vi "edit IPF.vi"(0 "New IPF":bool, 1 "Programs List":i32, 2 "APG Config":T6={"IPF Folder"=path "", "Results Folder"=path "", "Trace Folder"=path "", "a3DiCAD"={"Plot Spacing"=0.0, "TCF"=enum."STANDARD", "LeadLimit"=0, "a3DiCADDebug"=FALSE, "ODB"={"PrimePartNumber"=[], "SecondPartNumber"=[], "Height"={"PRP_CMP"="", "HEIGHT"=""}, "Units"={"PRP_CMP"="", "UNITS"=""}}, "PasteHeight"=0.0, "Inspection Performance"=TRUE}, "a3DiCADcfg"=path "", "Board Library"={"Board Library file"=path "", "Board library model folder"=path "", "Not Fittted/Fitted Components"=path "", "Panel Picture File"=path "", "Components"=enum."Fitted"}, "Site Library"={"Site Library file"=path "", "Site library model folder"=path ""}, "System Library"={"System Library file"=path "", "System library model folder"=path ""}, "ODB++ file"=path "", "Side ID Alias"={"Top"="", "Bottom"=""}}, 3 "Dongle Fitted event Refnum in":T1, 5 "error in":errorcluster, 6 "Main VI":refnum<vi>) -> (14 "Dongle fitted":bool, 16 "Program Name":string, 19 "error out":errorcluster)   [LabVIEW 2013, in "Manipulate IPF.lvlib"]
uses:
  Manipulate IPF.lvlib
  type_def/but_back.ctl
  3013/code/Modules/Configuration/type_def/Scan Params.ctl
  3013/code/Modules/Configuration/type_def/Profile Resolution.ctl
  3013/code/Modules/Preprocess Data/type_def/direction.ctl
  3013/code/Modules/GUI/GUI_5/subPanels/edit/type_def/GUI PCB List.ctl
  3013/code/Modules/Inspection/Data/PCB_class/type_def/PCB Params.ctl
  3013/code/Modules/Inspection/type_def/Pos and Rot.ctl
  3013/code/Modules/Barcode Reader/type_def/id.ctl
  3013/code/Modules/GUI/GUI_5/subPanels/edit/type_def/GUI Panel Params.ctl
  3013/code/Modules/Inspection/type_def/Range Limits.ctl
  3013/code/Modules/GUI/GUI_5/subPanels/edit/type_def/Description.ctl
  Settings/type_def/APG Config.ctl
  type_def/but_debug.ctl
  type_def/but_update TCF.ctl
  type_def/but_test coverage.ctl
  type_def/but_generate_Library_from TCF.ctl
  type_def/Dongle fitted event refnum.ctl
  type_def/state.ctl
  type_def/files.ctl
  3013/code/Modules/Inspection/Data/Panel_class/type_def/Config File data.ctl
  3013/code/Modules/Inspection/Data/Panel_class/type_def/BarCode Params.ctl
  3013/code/Modules/GUI/GUI_5/subPanels/edit/type_def/data.ctl
  3013/code/Modules/Inspection/Data/Panel_class/type_def/inspection data.ctl
  <vilib>/Utility/miscctls.llb/LVFontTypeDef.ctl
  type_def/Picture FGV commands.ctl
  Pack Data/type_def/file types.ctl
  type_def/IPF cmd.ctl
  <userlib>/_OpenG.lib/file/file.llb/Convert File Extension (Path)__ogtk.vi
  <userlib>/_OpenG.lib/file/file.llb/Strip Path Extension - 1D Array of Strings__ogtk.vi
  <userlib>/_OpenG.lib/file/file.llb/File Exists - Scalar__ogtk.vi
  <vilib>/Utility/cursorutil.llb/Set Cursor (Icon Pict).vi
  a3Di APG.lvlib
  3013/code/Modules/Inspection/Inspection.lvlib
  3013/code/Modules/Inspection/Data/PCB_class/PCB.lvclass
  3013/code/Modules/Barcode Reader/Barcode Reader.lvlib
  3013/code/Modules/Inspection/Data/Panel_class/Panel.lvclass
  3013/code/Modules/GUI/GUI_5/subPanels/edit/edit.lvlib
  3013/code/Modules/Preprocess Data/PreProcess.lvlib
  3013/code/Modules/Configuration/Config.lvlib
  Debug Results/Debug Results.lvlib
  3013/code/a3Di.lvlib
  Pack Data/Pack Files.lvlib
  3013/code/Modules/Inspection/Data/Fiducial_class/Fiducial.lvclass
  Mike/APG_mike a3Di.lvlib
  Update TCF/TCF update.lvlib
  Settings/APG_settings.lvlib
panel:
  in  "Side ID":string(combo)
  in  "Product Code":string
  in  "Initial Scan Button":bool caption="Initial Scan"
  in  "Generate Library button":T2
  in  "Test Coverage Button":T3
  in  "Update CAD Picture":bool
  in  "Delete CAD Picture":bool
  out "Panel Picture File":string
  in  "Update TCF button":T4
  out "PCB Outline File":string
  out "Control File":string
  out "Checking results":string
  in  "Debug Results Button":T5
  in  "Start Conversion ODB++":bool
  in  "Robot Scan Direction":enum32{"X", "Y", "X and Y"}(radio)
  in  "Add Fiducial":bool
  in  "Add PCB":bool
  in  "butReload":bool
  in  "butSave":bool
  in  "Description":T7
  in  "Fiducial List":T10(array[cluster]) {"Fiducial"."Pos & Rot"."Y" format="%#_8g"; "Fiducial"."Pos & Rot"."X" format="%#_8g"}
  in  "PCBs List":T11 {"PCB Params"."Pos & Rot"."Y" format="%#_8g"; "PCB Params"."Pos & Rot"."X" format="%#_8g"}
  in  "Panel Parameters":T14 {"Pos & Rot"."rotation" format="%#.3g"; "Pos & Rot"."Y" format="%#.3g"; "Pos & Rot"."X" format="%#.3g"}
  in  "Scan Params":T15={"Size of Scanning Area"={"x"=164.0, "y"=70.0}, "Scan Offset"={"x"=164.0, "y"=70.0}, "Slice Step in mm"=10.0, "Triggering Distance in mm"=0.0, "Triggering Distance in um"=0.0, "Profile Resolution"=enum."20 um", "Version"="", "Robot Scan Direction"=enum."X", "Initial scan"=FALSE}
  out "Program Name":string
  in  "Back Button":T18
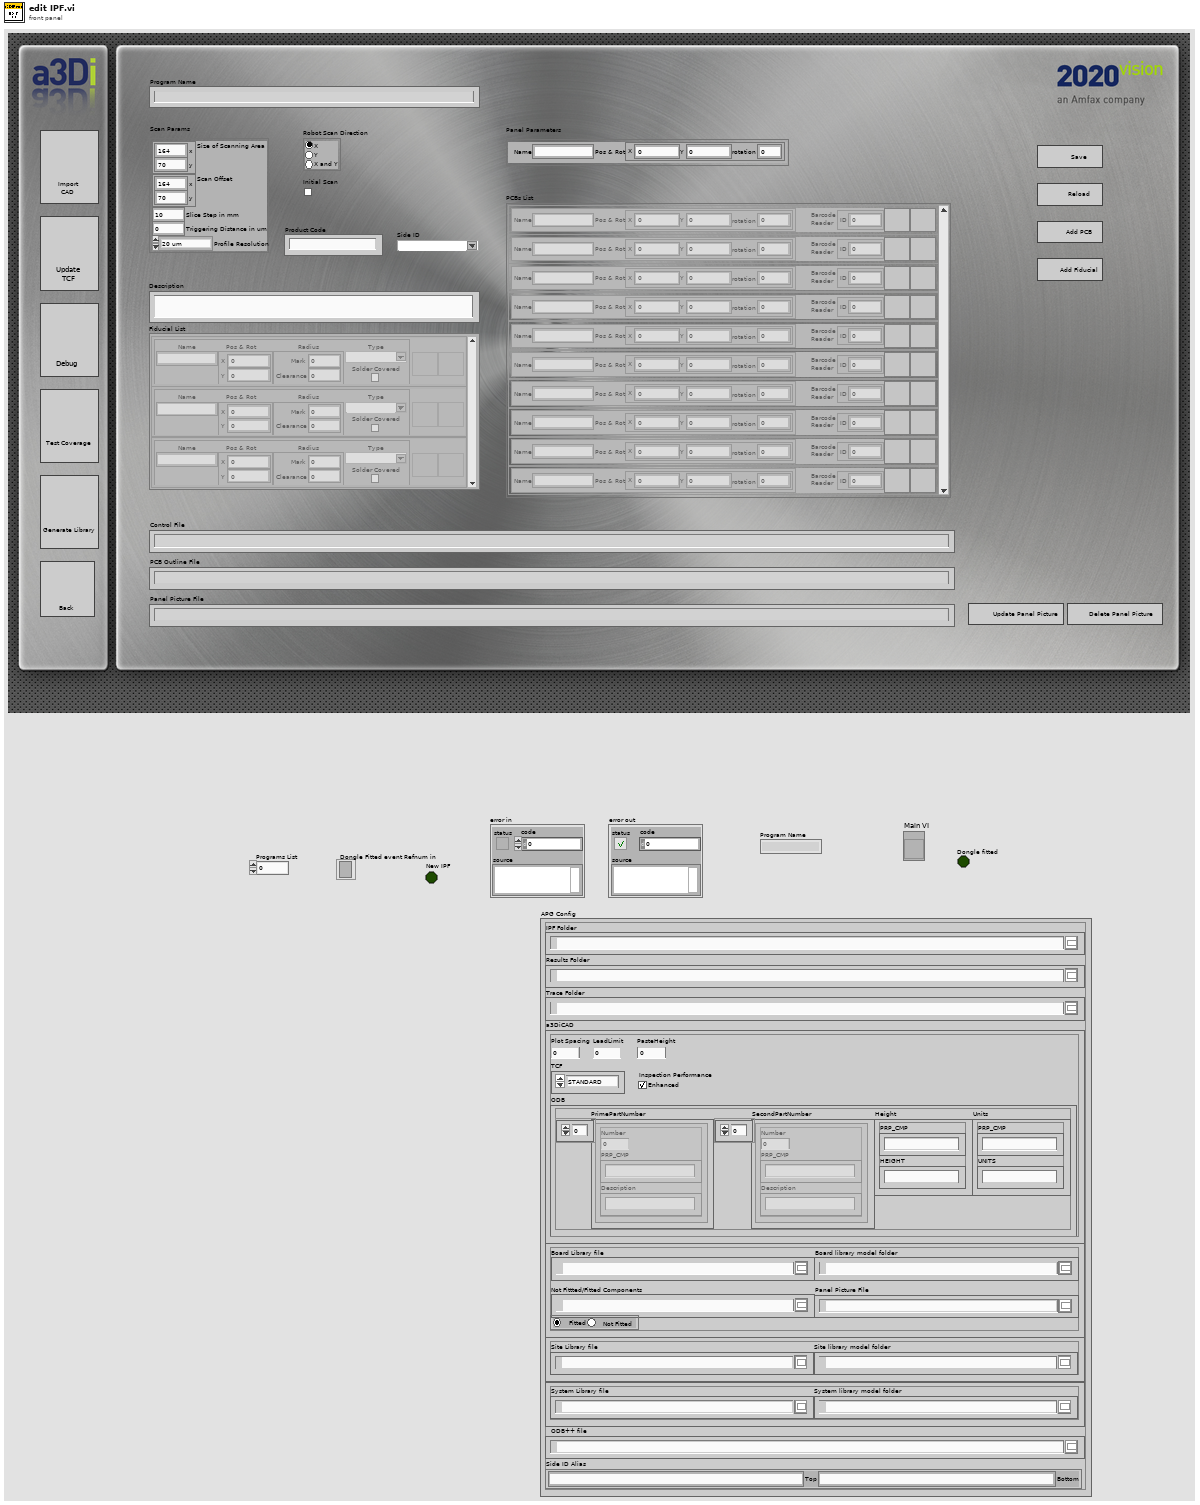
[diagram p1: front panel]
types:
  T1 = typedef "Dongle fitted event refnum.ctl" = refnum<event-registration>
  T2 = typedef "but_generate_Library_from TCF.ctl" = bool
  T3 = typedef "but_test coverage.ctl" = bool
  T4 = typedef "a3Di APG.lvlib/but_update TCF.ctl" = bool
  T5 = typedef "but_debug.ctl" = bool
  T6 = typedef "APG_settings.lvlib/APG Config.ctl" = cluster{"IPF Folder":path, "Results Folder":path, "Trace Folder":path, "a3DiCAD":cluster{"Plot Spacing":dbl, "TCF":enum16{"STANDARD", "PASTE", "LEAD"}, "LeadLimit":u32, "a3DiCADDebug":bool, "ODB":cluster{"PrimePartNumber":cluster{"Number":u32, "PRP_CMP":string, "Description":string}[], "SecondPartNumber":cluster{"Number":u32, "PRP_CMP":string, "Description":string}[], "Height":cluster{"PRP_CMP":string, "HEIGHT":string}, "Units":cluster{"PRP_CMP":string, "UNITS":string}}, "PasteHeight":dbl, "Inspection Performance":bool}, "a3DiCADcfg":path, "Board Library":cluster{"Board Library file":path, "Board library model folder":path, "Not Fittted/Fitted Components":path, "Panel Picture File":path, "Components":enum32{"Fitted", "Not Fitted "}}, "Site Library":cluster{"Site Library file":path, "Site library model folder":path}, "System Library":cluster{"System Library file":path, "System library model folder":path}, "ODB++ file":path, "Side ID Alias":cluster{"Top":string, "Bottom":string}}
  T7 = typedef "Description.ctl" = string
  T8 = typedef "Inspection.lvlib/Pos and Rot.ctl" = cluster{"X":dbl, "Y":dbl, "Z":dbl, "rotation":dbl}
  T9 = typedef "Inspection.lvlib/Range Limits.ctl" = cluster{"upper":sgl, "lower":sgl}
  T10 = cluster{"Fiducial":cluster{"Name":string, "Pos & Rot":T8, "Radius":cluster{"Mark":dbl, "Clearance":dbl}, "Inspection Params":cluster{"Clearance vs\nPad Threshold":dbl, "Avg Plane Limits":T9, "Edge Limit":T9}, "Type":string, "Solder Covered":bool}, "insert":bool, "delete":bool}[]
  T11 = typedef "GUI.lvlib/subPanel.lvlib/edit.lvlib/GUI PCB List.ctl" = cluster{"PCB Params":T12, "Barcode\nReader":cluster{"ID":T13}, "insert":bool, "delete":bool}[]
  T12 = typedef "Inspection.lvlib/PCB.lvclass/PCB Params.ctl" = cluster{"Name":string, "Pos & Rot":T8}
  T13 = typedef "Barcode Reader.lvlib/id.ctl" = u8
  T14 = typedef "GUI.lvlib/subPanel.lvlib/edit.lvlib/GUI Panel Params.ctl" = cluster{"Name":string, "Pos & Rot":T8}
  T15 = typedef "Config.lvlib/Scan Params.ctl" = cluster{"Size of Scanning Area":cluster{"x":dbl, "y":dbl}, "Scan Offset":cluster{"x":dbl, "y":dbl}, "Slice Step in mm":dbl, "Triggering Distance in mm":dbl, "Triggering Distance in um":dbl, "Profile Resolution":T16, "Version":string, "Robot Scan Direction":T17, "Initial scan":bool}
  T16 = typedef "Config.lvlib/Profile Resolution.ctl" = enum8{"20 um", "40 um"}
  T17 = typedef "PreProcess.lvlib/direction.ctl" = enum8{"X", "Y"}
  T18 = typedef "a3Di APG.lvlib/but_back.ctl" = bool
  T19 = typedef "GUI.lvlib/subPanel.lvlib/edit.lvlib/data.ctl" = cluster{"Program Name":string, "Scan Params[]":T15[], "Panel Params":T20, "Inspection Data":T22, "Control File Relative Path":path, "Description":string, "PCB Outline File":path, "Scan Start Delay":dbl, "CAD Picture File":string, "Product Code":string, "Side ID":string}
  T20 = typedef "Inspection.lvlib/Panel.lvclass/Config File data.ctl" = cluster{"Name":string, "Pos & Rot":T8, "PCBs List":cluster{"PCB Params":T12}[], "PCB BarCode Params":T21[], "Scan Type":bool}
  T21 = typedef "Inspection.lvlib/Panel.lvclass/BarCode Params.ctl" = cluster{"ID":T13}
  T22 = typedef "Inspection.lvlib/Panel.lvclass/inspection data.ctl" = cluster{"Fiducial List":cluster{"Name":string, "Position and Rotation":T8, "Radius":cluster{"Mark":dbl, "Clearance":dbl}, "Inspection Params":cluster{"Clearance vs Pad\nThreshold":dbl, "Avg Plane Limits":T9, "Edge Limit":T9}, "Type":string, "Solder Covered":bool}[]}
  T23 = typedef "a3Di APG.lvlib/files.ctl" = cluster{"Programming Files":cluster{"PCB Design Identity":string, "ODB++ file":path, "Result temp  folder":path, "IPF temp folder":path}, "ODB file Converted?":bool, "Panel Params":T20, "PCB Outline File":path, "Initial Scan":bool, "PCBs on a carrier":bool, "Carrier Size":cluster{"X":dbl, "Y":dbl}, "IPF modified":bool, "PCB Side":enum16{"Top", "Bottom"}}
  T24 = typedef "Manipulate IPF.lvlib/state.ctl" = enum16{"Initialise Inspection Program", "Wait for user input", "exit"}
  T25 = typedef "Manipulate IPF.lvlib/Picture FGV commands.ctl" = enum16{"No Action", "Set Update Picture", "Set Delete Picture", "Get Picture action"}
  T26 = typedef "LVFontTypeDef.ctl" = cluster{"Font Name":string, "Size":u16, "Bold":bool, "Italic":bool, "Underline":bool, "Strikeout":bool, "Color":u32}
  T27 = enum8{"Enabled", "Disabled", "Disabled and Grayed Out"}
  T28 = typedef "Pack Files.lvlib/file types.ctl" = enum16{"ODB", "TCF", "CAD Outline", "Config", "Inspection Prog", "a3Di-bin", "Results", "CAD Labels", "CAD Pads", "calScan_fid", "calScan_cal-tab", "PCB_SerialNumber", "CAD_Assembly", "Version", "Old Results", "CAD Picture", "Old TCF"}
  T29 = typedef "Manipulate IPF.lvlib/IPF cmd.ctl" = enum16{"New IPF", "Edit IPF", "Copy IPF", "Rename IPF", "Delete IPF", "Reload IPF", "Load all IPF"}
  T30 = cluster{"Debug Results Button":refnum<vi>, "insert":refnum<vi>, "Update TCF button":refnum<vi>, "delete":refnum<vi>, "Test Coverage Button":refnum<vi>, "PCBs List":refnum<vi>, "Fiducial List":refnum<vi>, "Scan Params":refnum<vi>, "Generate Library Button":refnum<vi>}
  T31 = cluster{"PCB Params":T12, "Barcode\nReader":cluster{"ID":T13}, "insert":bool, "delete":bool}
  T32 = cluster{"Fiducial":cluster{"Name":string, "Pos & Rot":T8, "Radius":cluster{"Mark":dbl, "Clearance":dbl}, "Inspection Params":cluster{"Clearance vs\nPad Threshold":dbl, "Avg Plane Limits":T9, "Edge Limit":T9}, "Type":string, "Solder Covered":bool}, "insert":bool, "delete":bool}
  T33 = cluster{"Name":string, "Pos & Rot":T8, "Radius":cluster{"Mark":dbl, "Clearance":dbl}, "Inspection Params":cluster{"Clearance vs\nPad Threshold":dbl, "Avg Plane Limits":T9, "Edge Limit":T9}, "Type":string, "Solder Covered":bool}
  T34 = typedef "Manipulate IPF.lvlib/Picture FGV actions.ctl" = enum16{"No Action", "Update Picture", "Delete Picture"}
  T35 = cluster{"PCB Params":cluster{"Name":bool, "Pos & Rot":cluster{"X":bool, "Y":bool, "Z":bool, "rotation":bool}}, "Barcode\nReader":cluster{"ID":bool}, "insert":bool, "delete":bool}[]
  T36 = cluster{"Fiducial":cluster{"Name":bool, "Pos & Rot":cluster{"X":bool, "Y":bool, "Z":bool, "rotation":bool}, "Radius":cluster{"Mark":bool, "Clearance":bool}, "Inspection Params":cluster{"Clearance vs\nPad Threshold":bool, "Avg Plane Limits":cluster{"upper":bool, "lower":bool}, "Edge Limit":cluster{"upper":bool, "lower":bool}}, "Type":bool, "Solder Covered":bool}, "insert":bool, "delete":bool}[]
  T37 = enum16{"Left", "Centre Left", "Centre Right", "Right", "Panel Close"}
  T38 = typedef "GUI.lvlib/subPanel.lvlib/edit.lvlib/GUI Panel & PCB params.ctl" = cluster{"Panel Params":T14, "PCBs List":T11}
  T39 = typedef "GUI.lvlib/subPanel.lvlib/edit.lvlib/GUI Fiducial List.ctl" = cluster{"Fiducial":cluster{"Name":string, "Pos & Rot":T8, "Radius":cluster{"Mark":dbl, "Clearance":dbl}, "Inspection Params":cluster{"Clearance vs\nPad Threshold":dbl, "Avg Plane Limits":T9, "Edge Limit":T9}, "Type":string, "Solder Covered":bool}, "insert":bool, "delete":bool}[]
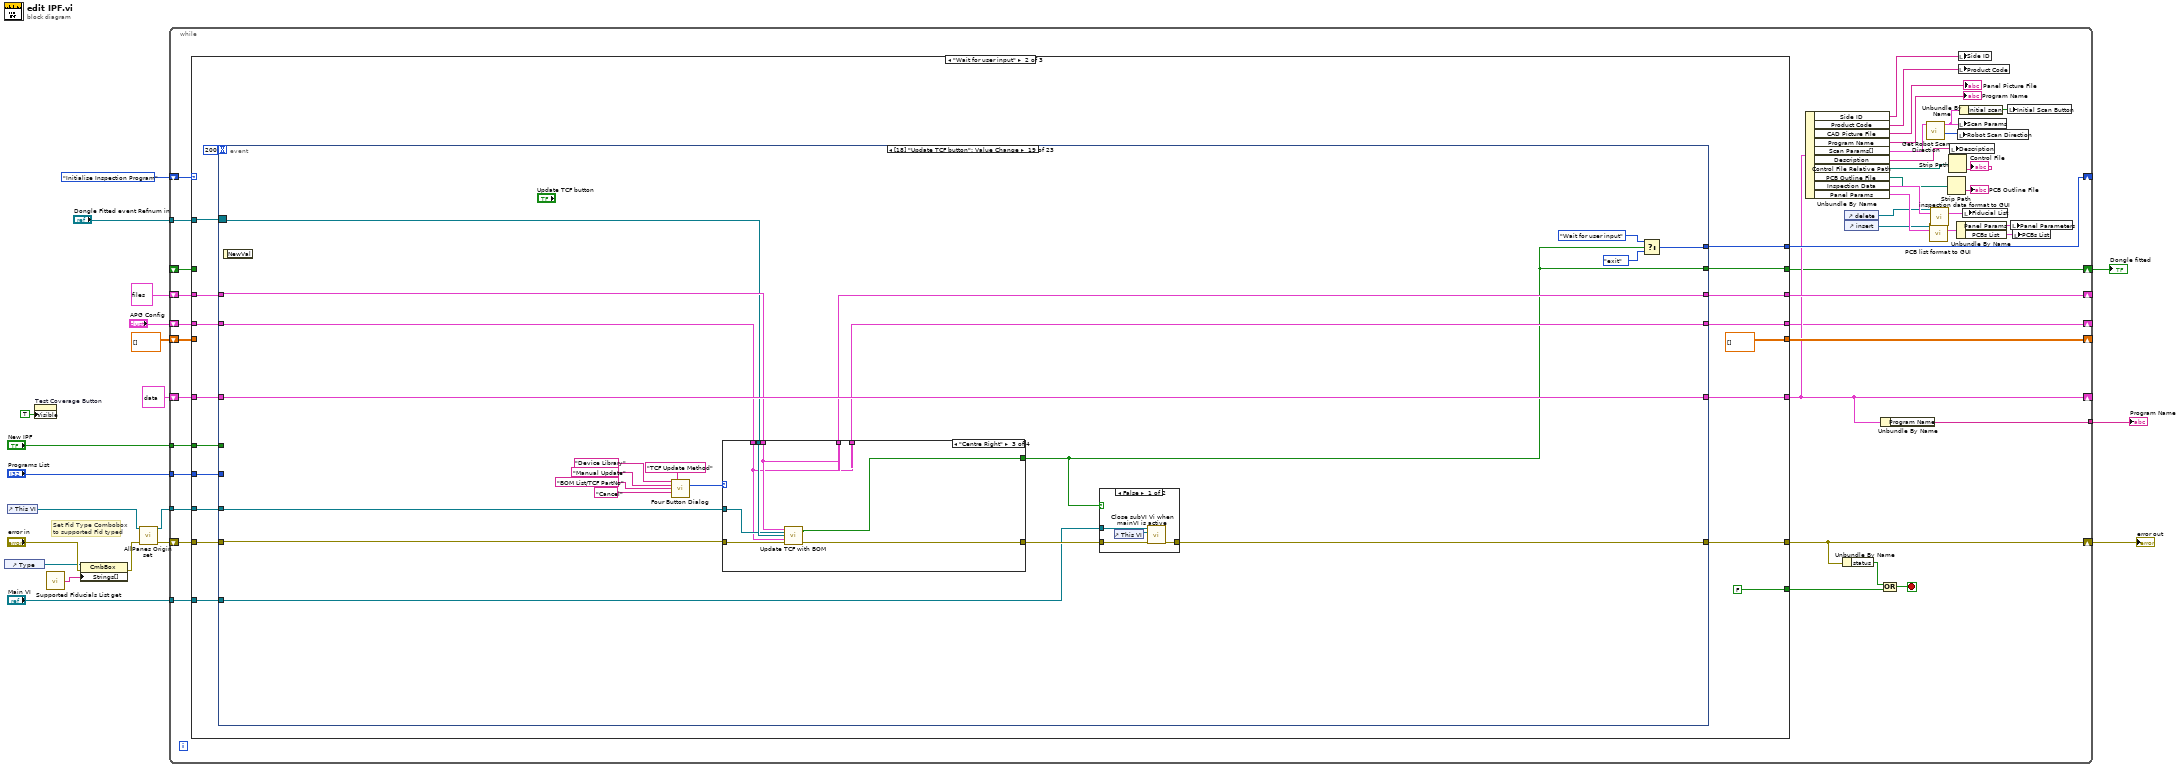
[diagram p0: block diagram]
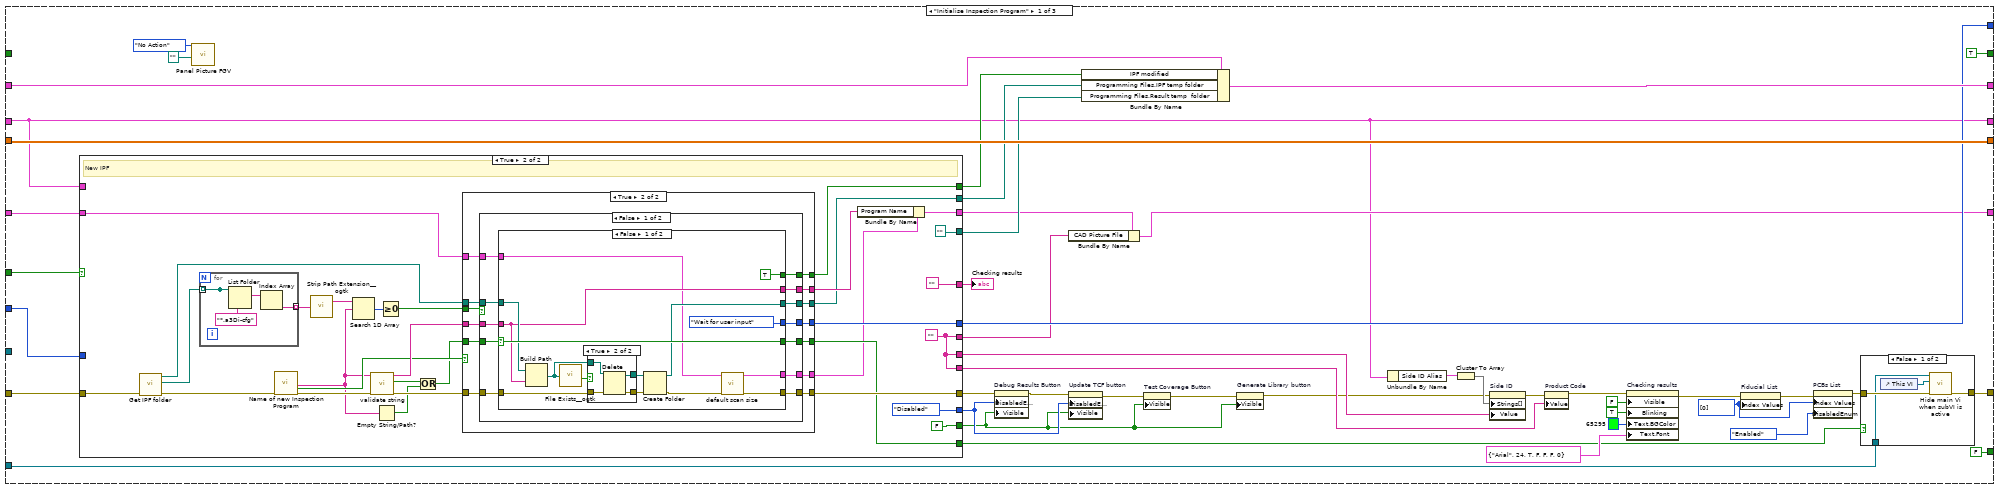
[diagram p2: hidden frame]
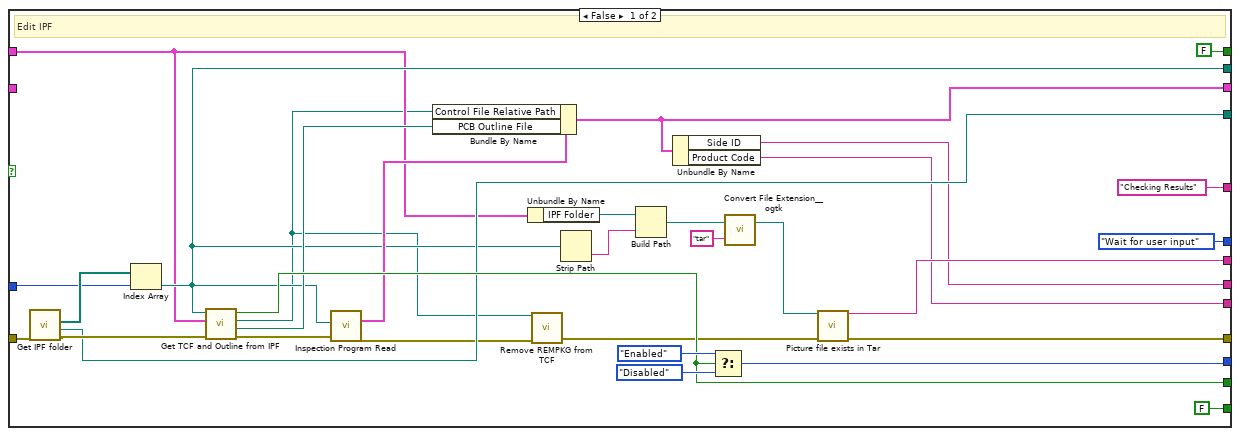
[diagram p4: hidden frame]
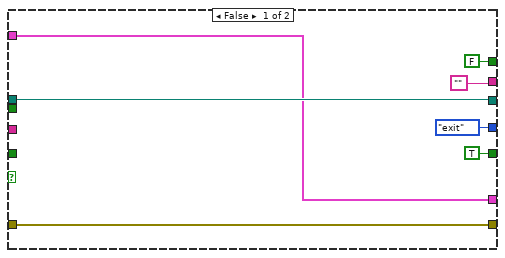
[diagram p5: hidden frame]
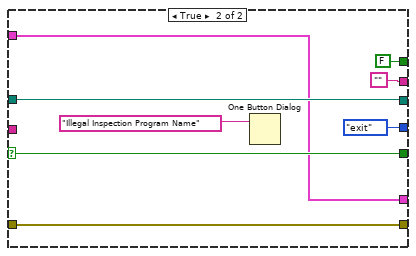
[diagram p7: hidden frame]
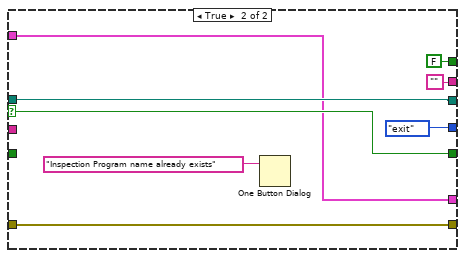
[diagram p8: hidden frame]
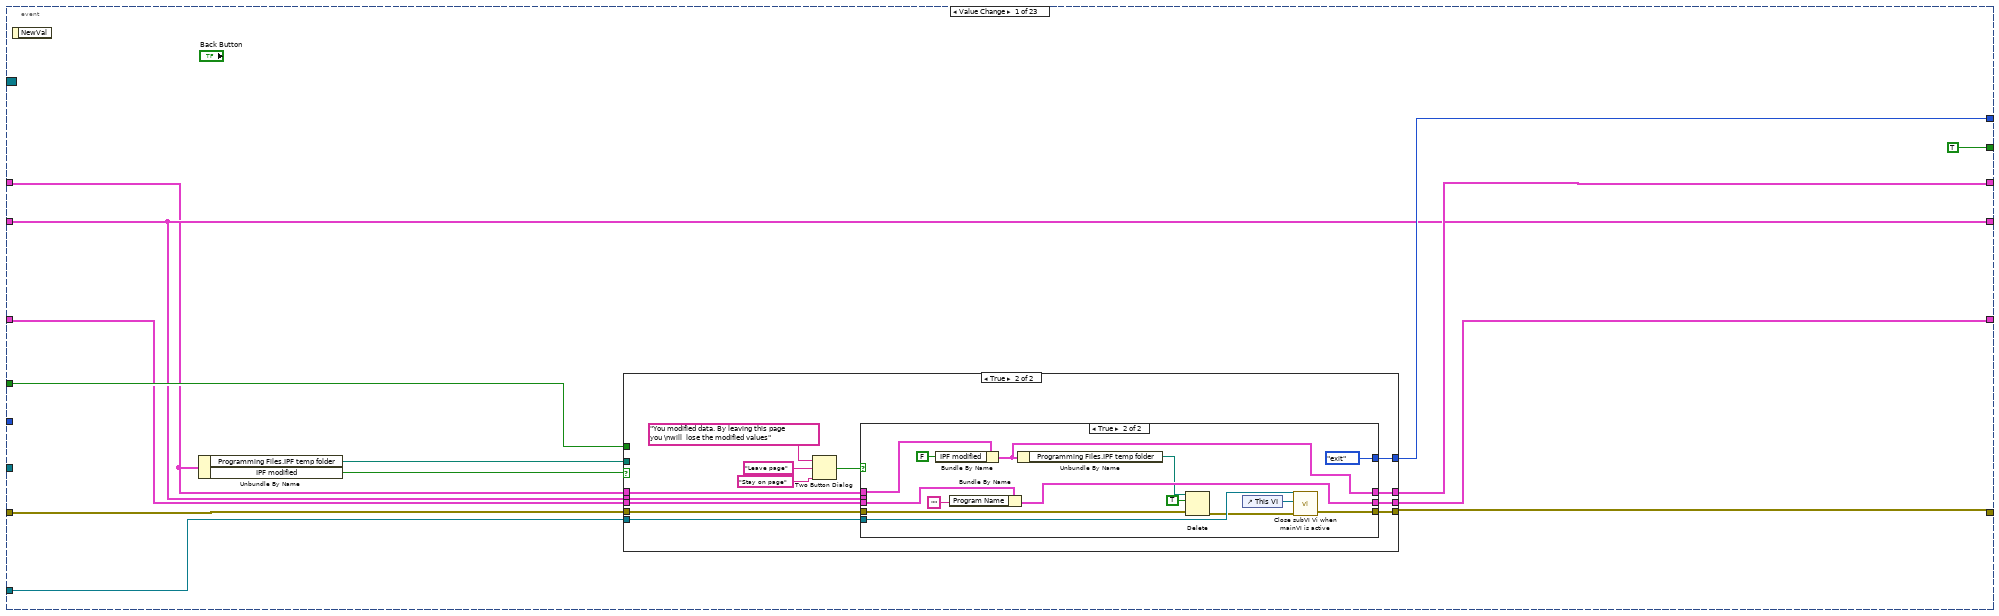
[diagram p9: hidden frame]
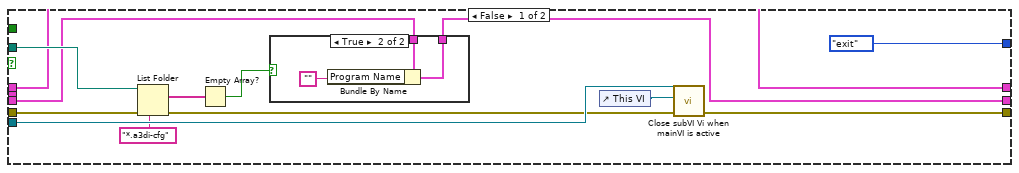
[diagram p10: hidden frame]
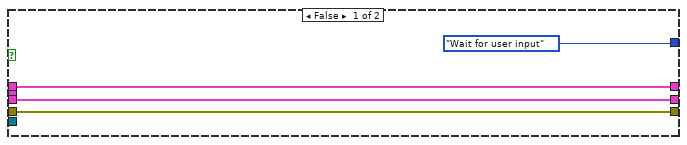
[diagram p12: hidden frame]
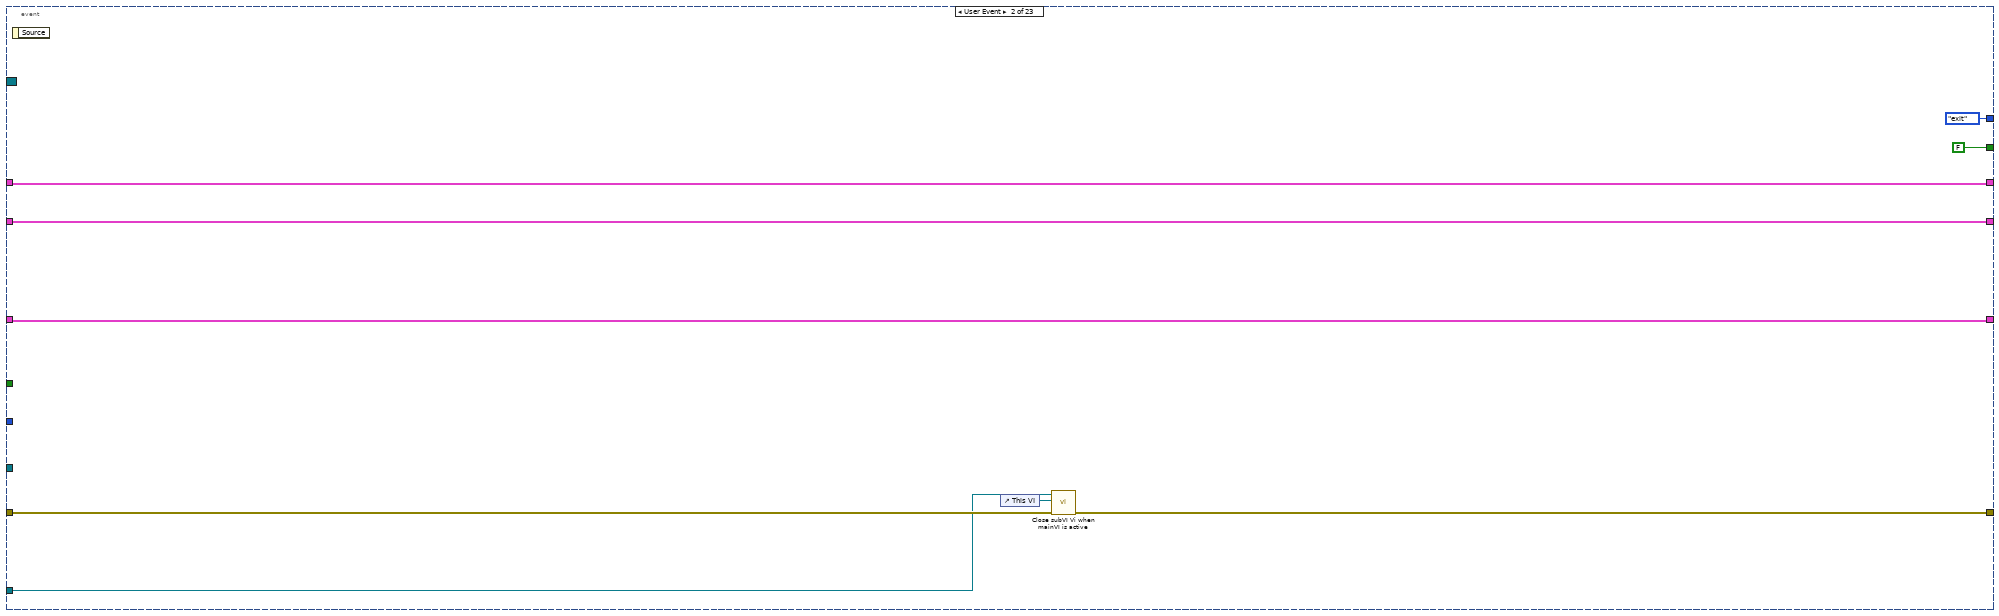
[diagram p13: hidden frame]
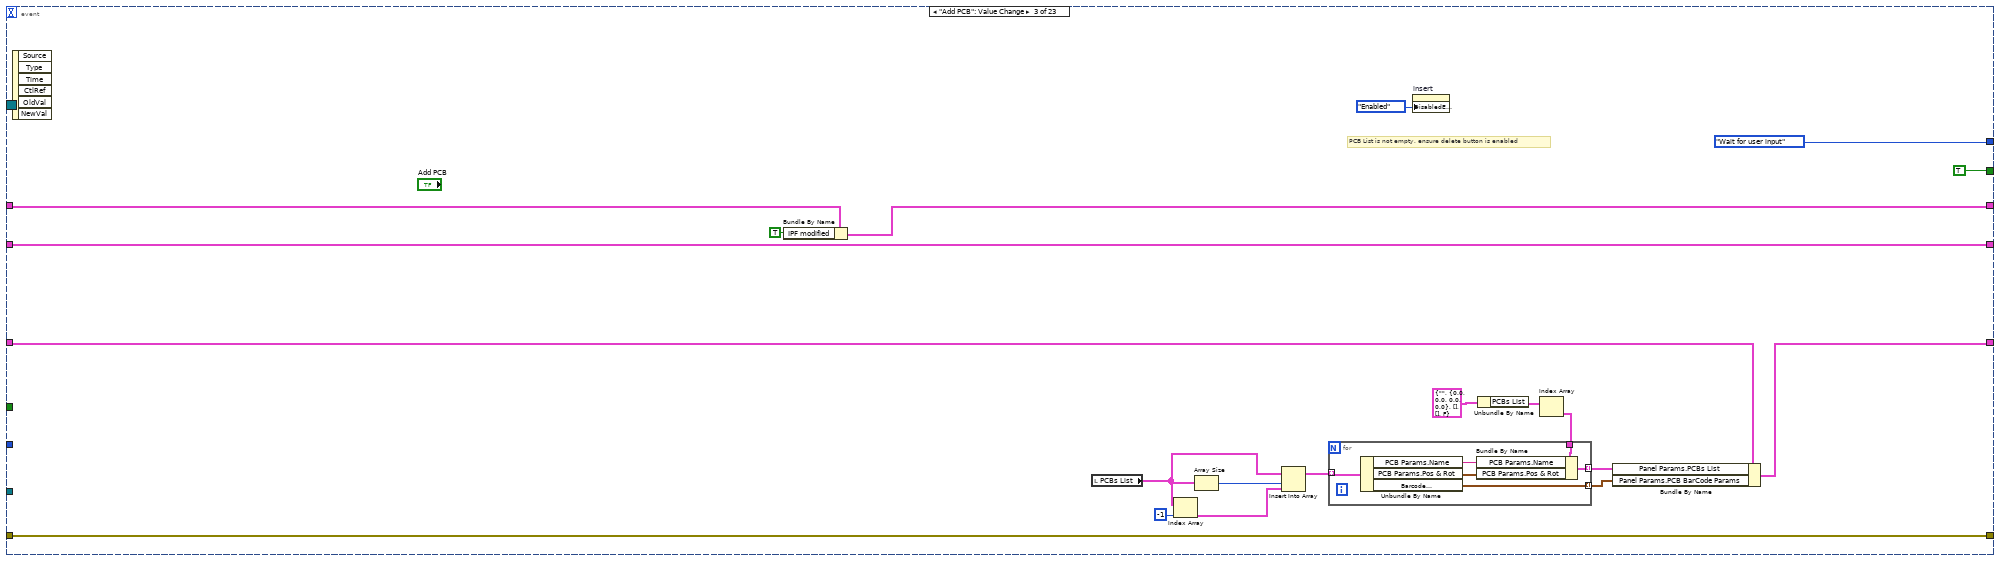
[diagram p14: hidden frame]
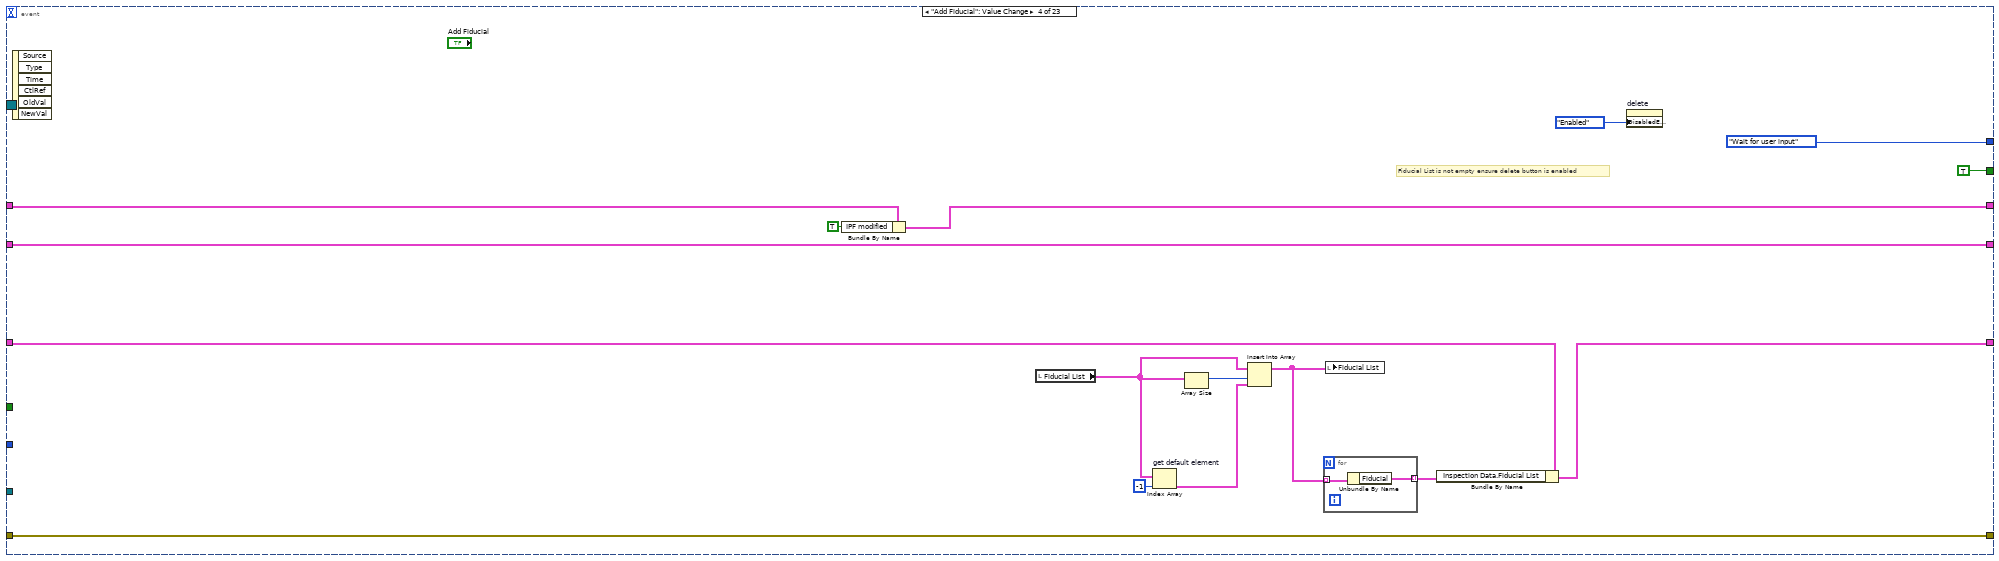
[diagram p15: hidden frame]
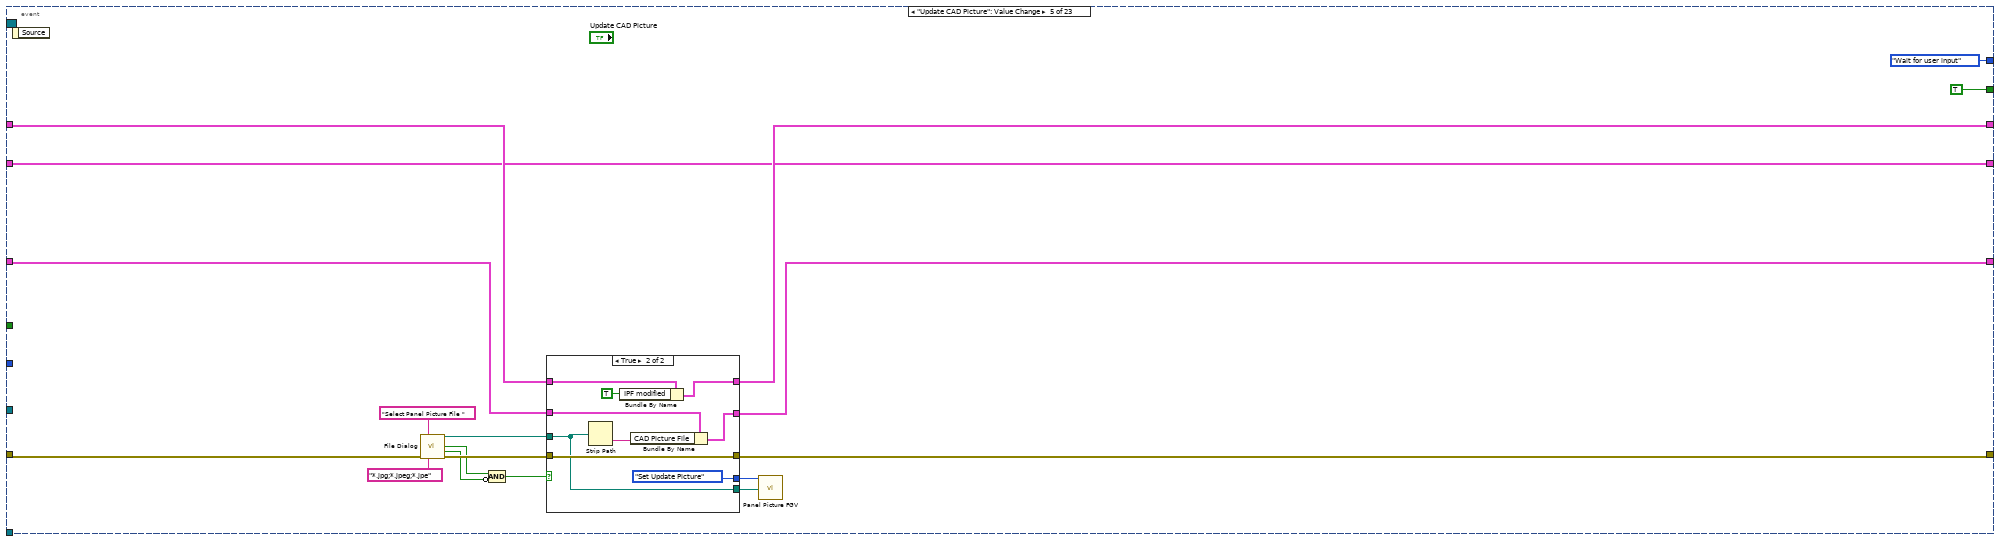
[diagram p16: hidden frame]
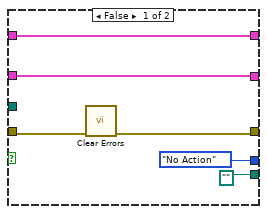
[diagram p17: hidden frame]
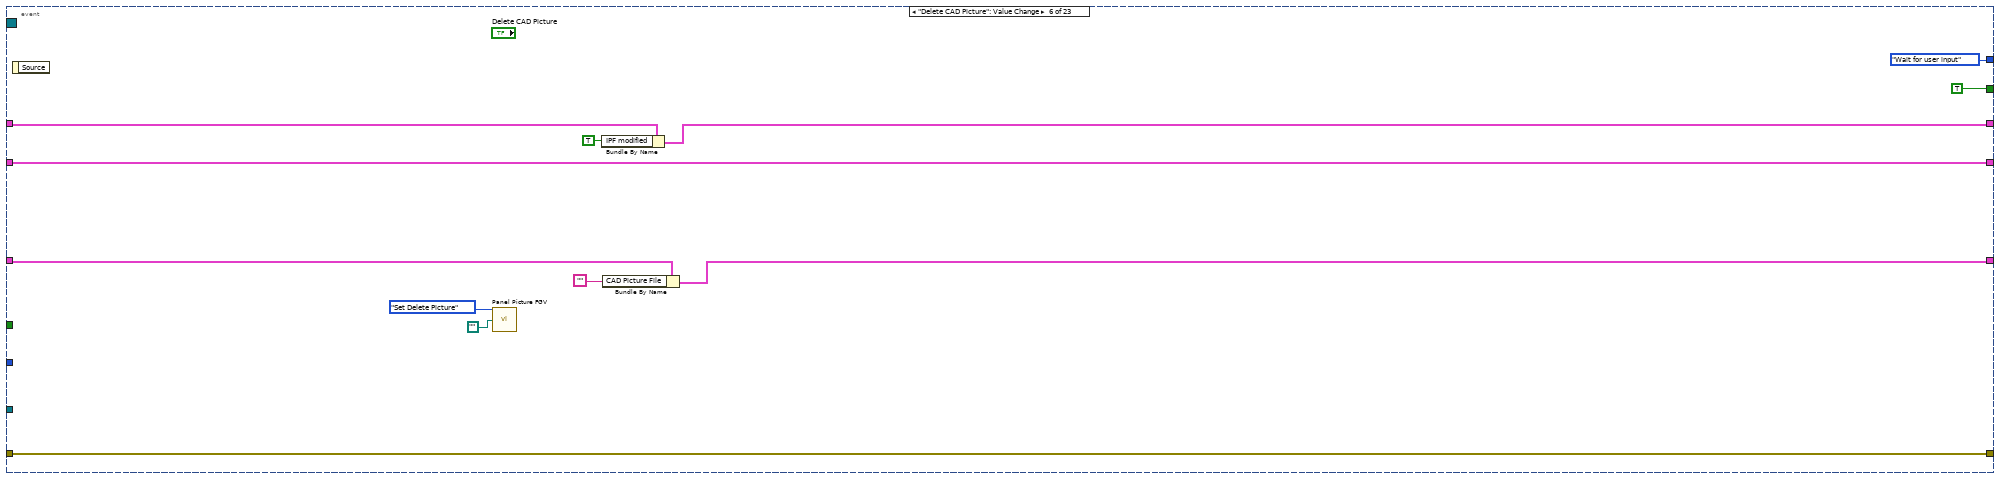
[diagram p18: hidden frame]
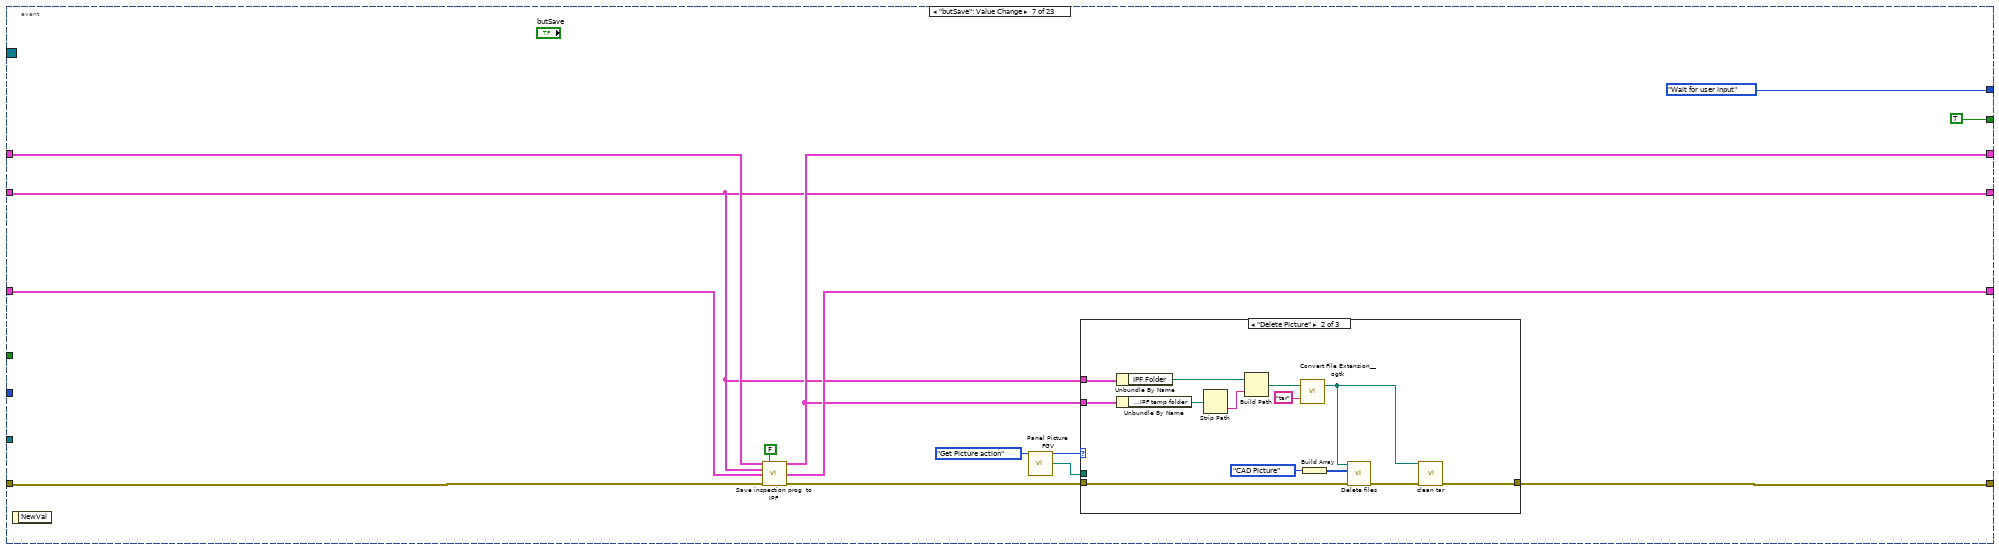
[diagram p19: hidden frame]
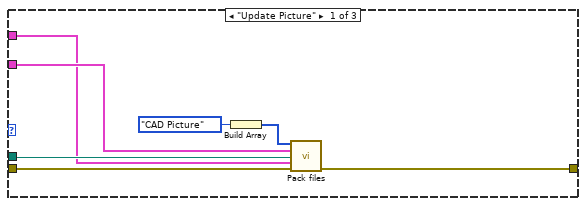
[diagram p20: hidden frame]
diagram:
  # "Set Fid Type Combobox\nto supported Fid typed"
  n1 = control-ref of="Type"() -> (w3:refnum<vi>)
  n2 = control-ref of="This VI"() -> (w6:refnum<vi>)
  n3 = property on="Test Coverage Button" class="Bool"("Visible"=TRUE) -> ()  [unwired: 2 in, 2 out]
  n4 = call "Supported Fiducials List get.vi"() -> ("Supported Fiducials[]"=w9:string[])  [unwired: 15 in]
  n5 = property class="CmbBox"(reference=w3, error in="error in", "Strings[]"=w9) -> (error out=w8:errorcluster)  [unwired: 1 out]
  n6 = call "AllPanes Origin set.vi"("VI ref in"=w6, "error in"=w8) -> ("VI ref out"=w5:refnum<vi>, "error out"=w20:errorcluster)  [unwired: 12 in]
  n7 = while {
    shift-right: [w63] -> _
    shift-left: state."Initialise Inspection Program" ("state") -> [w64]
    shift-right: [w59] -> w17
    shift-left: w20 -> [w62]
    shift-right: [w56] -> _
    shift-left: T23 {"Programming Files"={"PCB Design Identity"="", "ODB++ file"=path "", "Result temp  folder"=path "", "IPF temp folder"=path ""}, "ODB file Converted?"=FALSE, "Panel Params"={"Name"="", "Pos & Rot"={"X"=0.0, "Y"=0.0, "Z"=0.0, "rotation"=0.0}, "PCBs List"=[], "PCB BarCode Params"=[], "Scan Type"=FALSE}, "PCB Outline File"=path "", "Initial Scan"=FALSE, "PCBs on a carrier"=FALSE, "Carrier Size"={"X"=0.0, "Y"=0.0}, "IPF modified"=FALSE, "PCB Side"=enum."Top"} ("Programming Data Out") -> [w61]
    shift-right: [w38] -> _
    shift-left: T19 {"Program Name"="", "Scan Params[]"=[], "Panel Params"={"Name"="", "Pos & Rot"={"X"=0.0, "Y"=0.0, "Z"=0.0, "rotation"=0.0}, "PCBs List"=[], "PCB BarCode Params"=[], "Scan Type"=FALSE}, "Inspection Data"={"Fiducial List"=[]}, "Control File Relative Path"=path "", "Description"="", "PCB Outline File"=path "", "Scan Start Delay"=0.0, "CAD Picture File"="", "Product Code"="", "Side ID"=""} ("data out") -> [w55]
    shift-right: [w45] -> _
    shift-left: sgl[][] [] ("Scan Out") -> [w44]
    tunnel: "New IPF" -> [w40]
    tunnel: "Programs List" -> [w39]
    tunnel: [w28] -> w11
    tunnel: w5 -> [w37]
    tunnel: "Main VI" -> [w36]
    shift-right: [w30] -> _
    shift-left: "APG Config" -> [w41]
    tunnel: "Dongle Fitted event Refnum in" -> [w23]
    shift-right: [w22] -> w1
    shift-left: _ -> [w21]
    stop <- w60 stop-if-true
    n8 = case shown="\"Wait for user input\"" w64 {
      tunnel: [FALSE FALSE TRUE] -> w57
      tunnel: [w94 w265 state."exit" ("state")] -> w63
      tunnel: w62 -> [w97 w264 w854]
      tunnel: [w96 w259 w854] -> w59
      tunnel: [w106 w261 w858] -> w56
      tunnel: w61 -> [w78 w263 w858]
      tunnel: w55 -> [w105 w262 w856]
      tunnel: [w87 w260 w856] -> w38
      tunnel: [w108 sgl[][] [] ("Scan Out") sgl[][] [] ("Scan Out")] -> w45
      tunnel: w44 -> [w108 _ _]
      tunnel: w41 -> [w67 w257 w853]
      tunnel: w40 -> [w104 w253 _]
      tunnel: w39 -> [w103 w256 _]
      tunnel: w37 -> [_ w255 _]
      tunnel: w36 -> [w95 w254 _]
      tunnel: [w67 w252 w853] -> w30
      tunnel: w23 -> [_ w250 _]
      tunnel: [TRUE w249 w852] -> w22
      tunnel: w21 -> [_ _ w852]
      frame "Initialise Inspection Program" {
        w80 = u32[] [0] ("Index Values")
        n9 = case shown="True" w104 {
          tunnel: w97 -> [w139 w175]
          tunnel: [w123 w166] -> w107
          tunnel: [w130 w170] -> w91
          tunnel: w105 -> [_ w152]
          tunnel: [w117 w174] -> w86
          tunnel: w103 -> [w144 _]
          tunnel: w67 -> [w121 _]
          tunnel: [w134 FALSE ("Results extracted?")] -> w74
          tunnel: [w143 T27."Disabled" ("Disabled")] -> w89
          tunnel: ["Checking Results" ("Checking results") ""] -> w100
          tunnel: [state."Wait for user input" ("state") w168] -> w94
          tunnel: [FALSE ("String Modified") w167] -> w93
          tunnel: [FALSE ("IPF saved") w165] -> w92
          tunnel: [w131 path ""] -> w88
          tunnel: [w129 w146] -> w85
          tunnel: [w116 w146] -> w72
          tunnel: [w115 w146] -> w69
          frame False {
            # "Edit IPF"
            n10 = call "Get IPF folder.vi"("error in (no error)"=w139) -> ("error out"=w138:errorcluster, "Results Folder"=w131:path, "IPF sub folders"=w145:path[])  [unwired: 5 in, 3 out]
            n11 = Index Array(array=w145, index=w144) -> (element=w123:path)
            n12 = call "Get TCF and Outline from IPF.vi"("error in (no error)"=w138, "APG Config"=w121, "IPF temp folder"=w123) -> ("error out"=w137:errorcluster, "Outline path"=w132:path, "TCF path"=w118:path, "TCF in IPF"=w134:bool)  [unwired: 5 in]
            n13 = call "Inspection Program Read.vi"("error in (no error)"=w137, "ISP folder"=w123) -> ("error out"=w120:errorcluster, "data out"=w133:T19)  [unwired: 8 in]
            n14 = Bundle By Name(cluster=w133, "Control File Relative Path"=w118, "PCB Outline File"=w132) -> (w117:T19)
            n15 = Unbundle By Name(w121) -> ("IPF Folder"=w127:path)
            n16 = call "Remove REMPKG from TCF.vi"("TCF in"=w118, "error in"=w120) -> ("error out"=w119:errorcluster)  [unwired: 12 in, 1 out]
            n17 = Strip Path(path=w123) -> (name=w126:string)  [unwired: 1 out]
            n18 = Build Path(base path=w127, name or relative path=w126) -> (appended path=w125:path)
            n19 = Unbundle By Name(w117) -> ("Side ID"=w116:string, "Product Code"=w115:string)
            n20 = Select(t=T27."Enabled" ("Disabled"), s=w134, f=T27."Disabled" ("Disabled")) -> (s? t:f=w143:T27)
            n21 = call-poly <userlib>:"Convert File Extension__ogtk.vi"("new ending (none)"="tar", "file name"=w125) -> ("new filename"=w122:path)  [unwired: 1 out]
            n22 = call "Picture file exists in Tar.vi"("a3Di  tar file"=w122, "error in (no error)"=w119) -> ("CAD Picture"=w129:string, "error out"=w130:errorcluster)  [unwired: 11 in, 1 out]
          }
          frame True {
            w146 = ""
            # "New IPF"
            n23 = call "Get IPF folder.vi"("error in (no error)"=w175) -> ("error out"=w157:errorcluster, "IPF sub folders"=w158:path[], "IPF Folder"=w156:path)  [unwired: 5 in, 3 out]
            n24 = for {
              tunnel: [w245] -> _ mode=indexing
              tunnel: [w246] -> w163 mode=indexing
              tunnel: w158 -> [w245] mode=indexing
              n25 = List Folder(path=w245, pattern="*.a3Di-cfg") -> (filenames=w248:string[])  [unwired: 2 in, 3 out]
              n26 = Index Array(array=w248) -> (element=w246:string)  [unwired: 1 in]
            }
            n27 = call "Name of new Inspection Program"("error in (no error)"=w157) -> ("Inspection program name"=w151:string, "OK"=w154:bool, "error out"=w159:errorcluster)  [unwired: 16 in]
            n28 = call-poly <userlib>:"Strip Path Extension__ogtk.vi"("paths"=w163) -> ("roots"=w162:string[])  [unwired: 1 out]
            n29 = Search 1D Array(1D array=w162, element=w151) -> (index of element=w161:i32)  [unwired: 1 in]
            n30 = call "validate string.vi"("error in (no error)"=w159, "String In"=w151) -> ("error out"=w155:errorcluster, "String Modified"=w149:bool, "Modified String"=w164:string)  [unwired: 6 in, 1 out]
            n31 = Empty String/Path?(string/path=w151) -> (empty?=w150:bool)
            n32 = Greater Or Equal To 0?(x=w161) -> (x >= 0?=w160:bool)
            n33 = Or(x=w149, y=w150) -> (x .or. y?=w148:bool)
            n34 = case shown="True" w154 {
              tunnel: w164 -> [_ w195]
              tunnel: w148 -> [_ w194]
              tunnel: w160 -> [_ w193]
              tunnel: [state."exit" ("state") w192] -> w168
              tunnel: [TRUE w191] -> w167
              tunnel: [FALSE ("IPF saved") w190] -> w165
              tunnel: w156 -> [w179 w189]
              tunnel: [w179 w188] -> w166
              tunnel: [w182 w187] -> w170
              tunnel: w155 -> [w182 w186]
              tunnel: ["" w185] -> w169
              tunnel: [w176 w184] -> w153
              tunnel: w152 -> [w176 w183]
              frame False {
              }
              frame True {
                n35 = case shown="False" w193 {
                  selector: w193 -> [_ w242]
                  tunnel: w195 -> [w207 _]
                  tunnel: [w206 ""] -> w185
                  tunnel: [w205 state."exit" ("state")] -> w192
                  tunnel: w194 -> [w204 _]
                  tunnel: [w203 w242] -> w191
                  tunnel: [w202 FALSE ("IPF saved")] -> w190
                  tunnel: w189 -> [w201 w240]
                  tunnel: [w200 w240] -> w188
                  tunnel: [w199 w239] -> w187
                  tunnel: w186 -> [w198 w239]
                  tunnel: [w197 w237] -> w184
                  tunnel: w183 -> [w196 w237]
                  frame False {
                    n36 = case shown="False" w204 {
                      selector: w204 -> [w221 w233]
                      tunnel: w207 -> [w217 _]
                      tunnel: [w217 ""] -> w206
                      tunnel: [state."Wait for user input" ("state") state."exit" ("state")] -> w205
                      tunnel: [w221 w233] -> w203
                      tunnel: [TRUE ("IPF saved") FALSE ("IPF saved")] -> w202
                      tunnel: w201 -> [w219 w231]
                      tunnel: [w218 w231] -> w200
                      tunnel: [w215 w230] -> w199
                      tunnel: w198 -> [w212 w230]
                      tunnel: [w214 w229] -> w197
                      tunnel: w196 -> [w213 w229]
                      frame False {
                        n37 = Build Path(base path=w219, name or relative path=w217) -> (appended path=w209:path)
                        n38 = call-poly <userlib>:"File Exists__ogtk.vi"("file path"=w209) -> ("exists"=w210:bool)  [unwired: 6 in, 1 out]
                        n39 = case shown="True" w210 {
                          tunnel: w212 -> [w224 w228]
                          tunnel: [w224 w227] -> w211
                          tunnel: w209 -> [w223 w226]
                          tunnel: [w223 w225] -> w208
                          frame False {
                          }
                          frame True {
                            n40 = Delete(path (use dialog)=w226, error in=w228) -> (deleted path=w225:path, error out=w227:errorcluster)  [unwired: 3 in, 1 out]
                          }
                        }
                        n41 = Create Folder(path (use dialog)=w208, error in=w211) -> (created path=w218:path, error out=w216:errorcluster)  [unwired: 1 in, 1 out]
                        n42 = call "default scan size.vi"("data in"=w213, "error in"=w216) -> ("data out"=w214:T19, "error out"=w215:errorcluster)  [unwired: 12 in]
                      }
                      frame True {
                        n43 = One Button Dialog(message="Illegal Inspection Program Name") -> ()  [unwired: 1 in, 1 out]
                      }
                    }
                  }
                  frame True {
                    n44 = One Button Dialog(message="Inspection Program name already exists") -> ()  [unwired: 1 in, 1 out]
                  }
                }
              }
            }
            n45 = Bundle By Name(cluster=w153, "Program Name"=w169) -> (w174:T19)
          }
        }
        "Checking results" <- w100
        n46 = call "Panel Picture FGV.vi"("Panel Picture Command"=Picture_FGV_commands."No Action", "Panel Picture path in"=path "") -> ()  [unwired: 12 in, 2 out]
        n47 = property on="Debug Results Button" class="Bool"(error in=w91, "DisabledEnum"=w89, "Visible"=w74) -> (error out=w90:errorcluster)  [unwired: 1 in, 1 out]
        n48 = Bundle By Name(cluster=w86, "CAD Picture File"=w85) -> (w87:T19)
        n49 = property on="Update TCF button" class="Bool"(error in=w90, "DisabledEnum"=w89, "Visible"=w74) -> (error out=w77:errorcluster)  [unwired: 1 in, 1 out]
        n50 = Bundle By Name(cluster=w78, "IPF modified"=w92, "Programming Files.IPF temp folder"=w107, "Programming Files.Result temp  folder"=w88) -> (w106:T23)
        n51 = property on="Test Coverage Button" class="Bool"(error in=w77, "Visible"=w74) -> (error out=w76:errorcluster)  [unwired: 1 in, 1 out]
        n52 = property on="Generate Library button" class="Bool"(error in=w76, "Visible"=w74) -> (error out=w68:errorcluster)  [unwired: 1 in, 1 out]
        n53 = Unbundle By Name(w67) -> ("Side ID Alias"=w66:cluster{"Top":string, "Bottom":string})
        n54 = Cluster To Array(cluster=w66) -> (array=w73:string[])
        n55 = property on="Side ID" class="CmbBox"(error in=w68, "Strings[]"=w73, "Value"=w72) -> (error out=w71:errorcluster)  [unwired: 1 in, 1 out]
        n56 = property on="Product Code" class="Str"(error in=w71, "Value"=w69) -> (error out=w70:errorcluster)  [unwired: 1 in, 1 out]
        n57 = property on="Checking results" class="Str"(error in=w70, "Visible"=FALSE, "Blinking"=TRUE, "Text.BGColor"=u32 65295, "Text.Font"=T26 {"Font Name"="Arial", "Size"=24, "Bold"=TRUE, "Italic"=FALSE, "Underline"=FALSE, "Strikeout"=FALSE, "Color"=0}) -> (error out=w82:errorcluster)  [unwired: 1 in, 1 out]
        n58 = property on="Fiducial List" class="Arr"(error in=w82, "Index Values"=w80) -> (error out=w81:errorcluster)  [unwired: 1 in, 1 out]
        n59 = property on="PCBs List" class="Arr"(error in=w81, "Index Values"=w80, "DisabledEnum"=T27."Enabled" ("Disabled")) -> (error out=w75:errorcluster)  [unwired: 1 in, 1 out]
        n60 = case shown="False" w93 {
          tunnel: [w113 w114] -> w96
          tunnel: w75 -> [w112 w114]
          tunnel: w95 -> [w111 _]
          frame False {
            n61 = control-ref of="This VI"() -> (w110:refnum<vi>)
            n62 = call "Hide main Vi when subVI is active.vi"("error in (no error)"=w112, "sub Vi ref"=w110, "Parent VI ref"=w111) -> ("error out"=w113:errorcluster)  [unwired: 8 in]
          }
          frame True {
          }
        }
      }
      frame "Wait for user input" {
        n63 = event shown="[18] \"Update TCF button\": Value Change" {
          selector: w250 -> [_ _ _ _ _ _ _ _ _ w504 _ _ _ _ _ _ w691 _ w743 w802 _ _ _]
          dyn-events: _ -> [_ _ _ _ _ _ _ _ _ _ _ _ _ _ _ _ _ _ _ _ _ _ _]
          timeout: 200 -> [_ _ _ _ _ _ _ _ _ _ _ _ _ _ _ _ _ _ _ _ _ _ _]
          tunnel: [w275 state."exit" ("state") state."Wait for user input" ("state") state."Wait for user input" ("state") state."Wait for user input" ("state") state."Wait for user input" ("state") state."Wait for user input" ("state") state."Wait for user input" ("state") state."Wait for user input" ("state") w501 state."Wait for user input" ("state") state."Wait for user input" ("state") state."Wait for user input" ("state") state."Wait for user input" ("state") state."Wait for user input" ("state") state."Wait for user input" ("state") w688 state."Wait for user input" ("state") w740 w799 state."Wait for user input" ("state") state."Wait for user input" ("state") state."Wait for user input" ("state")] -> w265
          tunnel: w264 -> [w279 w331 w342 w370 w396 w424 w438 w466 w483 w509 w524 w540 w546 w558 w618 w668 w698 w717 w728 w804 w816 w830 w846]
          tunnel: w263 -> [w270 w334 w340 w368 w386 w420 w437 w464 w488 w508 w519 w531 w544 w556 w616 w666 w694 w719 w744 w806 w820 w840 w848]
          tunnel: w262 -> [w269 w335 w345 w371 w395 w422 w436 w465 _ w510 w527 w534 w552 w561 w622 w672 w693 w718 w748 w803 w818 w837 w844]
          tunnel: [w278 w334 w339 w367 w385 w419 w429 w464 w487 w508 w518 w530 w543 w555 w615 w665 w696 w719 w746 w806 w821 w839 w847] -> w261
          tunnel: [w277 w335 w344 w372 w394 w421 w435 w465 w475 w510 w526 w537 w548 w565 w623 w670 w699 w718 w748 w803 w817 w836 w843] -> w260
          tunnel: [w273 w330 w342 w370 w397 w424 w430 w466 w479 w499 w524 w540 w546 w558 w618 w668 w686 w711 w738 w796 w816 w829 w846] -> w259
          tunnel: w257 -> [w271 w333 w338 w366 w382 w415 w427 w462 w468 w505 w517 w529 w542 w554 w614 w664 w697 w707 w745 w805 w819 w838 w850]
          tunnel: w256 -> [_ _ _ _ _ _ _ _ _ _ _ _ _ _ _ _ _ _ _ _ _ _ _]
          tunnel: w255 -> [_ _ _ _ _ _ _ _ _ _ _ _ _ _ _ _ w695 _ w735 _ _ _ _]
          tunnel: w254 -> [w274 w329 _ _ _ _ _ _ _ w498 _ _ _ _ _ _ w685 _ w737 w797 _ _ _]
          tunnel: w253 -> [w272 _ _ _ _ _ _ _ _ _ _ _ _ _ _ _ _ _ _ _ _ _ _]
          tunnel: [w271 w333 w338 w366 w382 w415 w427 w462 w468 w505 w517 w529 w542 w554 w614 w664 w692 w706 w747 w805 w819 w838 w850] -> w252
          tunnel: [TRUE FALSE TRUE TRUE TRUE TRUE TRUE TRUE TRUE w497 TRUE TRUE TRUE TRUE TRUE TRUE w684 TRUE w736 w795 TRUE TRUE TRUE] -> w249
          event Value Change {
            n64 = event-data() -> ()  [unwired: 1 in, 1 out]
            n65 = Unbundle By Name(w270) -> ("Programming Files.IPF temp folder"=w268:path, "IPF modified"=w276:bool)
            n66 = case shown="True" w276 {
              tunnel: w279 -> [w282 w309]
              tunnel: [w290 w308] -> w273
              tunnel: w270 -> [w280 w299]
              tunnel: w271 -> [_ w307]
              tunnel: w269 -> [w285 w306]
              tunnel: [w280 w305] -> w278
              tunnel: [w284 w304] -> w277
              tunnel: [state."exit" ("state") w298] -> w275
              tunnel: w274 -> [w289 w297]
              tunnel: w272 -> [_ _]
              tunnel: w268 -> [w286 _]
              frame False {
                n67 = List Folder(path=w286, pattern="*.a3di-cfg", error in=w282) -> (filenames=w288:string[], error out=w281:errorcluster)  [unwired: 1 in, 2 out]
                n68 = Empty Array?(array=w288) -> (empty?=w283:bool)
                n69 = case shown="True" w283 {
                  tunnel: w285 -> [w293 w295]
                  tunnel: [w293 w294] -> w284
                  frame False {
                  }
                  frame True {
                    n70 = Bundle By Name(cluster=w295, "Program Name"="") -> (w294:T19)
                  }
                }
                n71 = control-ref of="This VI"() -> (w291:refnum<vi>)
                n72 = call "Close subVI Vi when mainVI is active.vi"("error in (no error)"=w281, "Sub Vi ref"=w291, "Parent VI ref"=w289) -> ("error out"=w290:errorcluster)  [unwired: 8 in]
              }
              frame True {
                n73 = Two Button Dialog(message="You modified data. By leaving this page you \nwill  lose the modified values", 1:"Stay on page" ("F button name (\"Cancel\")"), 2:"Leave page" ("T button name (\"OK\")")) -> (T button?=w300:bool)
                n74 = case shown="True" w300 {
                  tunnel: w309 -> [w312 w318]
                  tunnel: [w312 w320] -> w308
                  tunnel: w299 -> [w311 w327]
                  tunnel: w307 -> [_ _]
                  tunnel: w306 -> [w310 w325]
                  tunnel: [w311 w316] -> w305
                  tunnel: [w310 w322] -> w304
                  tunnel: [state."Wait for user input" ("state") state."exit" ("state")] -> w298
                  tunnel: w297 -> [_ w319]
                  frame False {
                  }
                  frame True {
                    n75 = Bundle By Name(cluster=w327, "IPF modified"=FALSE) -> (w316:T23)
                    n76 = Bundle By Name(cluster=w325, "Program Name"="") -> (w322:T19)
                    n77 = Unbundle By Name(w316) -> ("Programming Files.IPF temp folder"=w315:path)
                    n78 = Delete(path (use dialog)=w315, entire hierarchy (F)=TRUE, error in=w318) -> (error out=w317:errorcluster)  [unwired: 2 in, 2 out]
                    n79 = control-ref of="This VI"() -> (w321:refnum<vi>)
                    n80 = call "Close subVI Vi when mainVI is active.vi"("error in (no error)"=w317, "Sub Vi ref"=w321, "Parent VI ref"=w319) -> ("error out"=w320:errorcluster)  [unwired: 8 in]
                  }
                }
              }
            }
          }
          event User Event {
            n81 = event-data() -> ()  [unwired: 1 in, 1 out]
            n82 = control-ref of="This VI"() -> (w332:refnum<vi>)
            n83 = call "Close subVI Vi when mainVI is active.vi"("error in (no error)"=w331, "Sub Vi ref"=w332, "Parent VI ref"=w329) -> ("error out"=w330:errorcluster)  [unwired: 8 in]
          }
          event "Add PCB": Value Change {
            # "PCB List is not empty, ensure delete button is enabled"
            n84 = event-data() -> ()  [unwired: 1 in, 6 out]
            n85 = Bundle By Name(cluster=w340, "IPF modified"=TRUE ("IPF saved")) -> (w339:T23)
            n86 = local read "PCBs List"() -> (w353:T11)
            n87 = Index Array(array=w353, index=-1) -> (element=w356:T31)
            n88 = Array Size(array=w353) -> (size(s)=w354:i32)
            n89 = Insert Into Array(array=w353, index=w354, new element=w356) -> (w346:T11)
            n90 = property on="insert" class="Bool"("DisabledEnum"=T27."Enabled" ("Disabled")) -> ()  [unwired: 2 in, 2 out]
            n91 = Unbundle By Name(T20 {"Name"="", "Pos & Rot"={"X"=0.0, "Y"=0.0, "Z"=0.0, "rotation"=0.0}, "PCBs List"=[], "PCB BarCode Params"=[], "Scan Type"=FALSE} ("Panel Params")) -> ("PCBs List"=w348:cluster{"PCB Params":T12}[])
            n92 = Index Array(array=w348) -> (element=w347:cluster{"PCB Params":T12})  [unwired: 1 in]
            n93 = for {
              tunnel: w346 -> [w362] mode=indexing
              tunnel: [w359] -> w350 mode=indexing
              tunnel: w347 -> [w358]
              tunnel: [w357] -> w343 mode=indexing
              n94 = Unbundle By Name(w362) -> ("PCB Params.Name"=w361:string, "PCB Params.Pos & Rot"=w360:T8, "Barcode\nReader"=w357:cluster{"ID":T13})
              n95 = Bundle By Name(cluster=w358, "PCB Params.Name"=w361, "PCB Params.Pos & Rot"=w360) -> (w359:cluster{"PCB Params":T12})
            }
            n96 = Bundle By Name(cluster=w345, "Panel Params.PCBs List"=w350, "Panel Params.PCB BarCode Params"=w343) -> (w344:T19)
          }
          event "Add Fiducial": Value Change {
            # "Fiducial List is not empty ensure delete button is enabled"
            n97 = event-data() -> ()  [unwired: 1 in, 6 out]
            n98 = Bundle By Name(cluster=w368, "IPF modified"=TRUE ("IPF saved")) -> (w367:T23)
            n99 = local read "Fiducial List"() -> (w374:T10)
            n100 = Index Array "get default element"(array=w374, index=-1) -> (element=w378:T32)
            n101 = Array Size(array=w374) -> (size(s)=w376:i32)
            n102 = Insert Into Array(array=w374, index=w376, new element=w378) -> (w373:T10)
            n103 = for {
              tunnel: w373 -> [w380] mode=indexing
              tunnel: [w379] -> w365 mode=indexing
              n104 = Unbundle By Name(w380) -> ("Fiducial"=w379:T33)
            }
            n105 = local write "Fiducial List"(w373) -> ()
            n106 = Bundle By Name(cluster=w371, "Inspection Data.Fiducial List"=w365) -> (w372:T19)
            n107 = property on="delete" class="Bool"("DisabledEnum"=T27."Enabled" ("Disabled")) -> ()  [unwired: 2 in, 2 out]
          }
          event "Update CAD Picture": Value Change {
            n108 = event-data() -> ()  [unwired: 1 in, 1 out]
            n109 = call "File Dialog"("prompt"="Select Panel Picture File ", "error in"=w396, "pattern (all files)"="*.jpg;*.jpeg;*.jpe") -> ("selected path"=w392:path, "exists"=w389:bool, "cancelled"=w387:bool, "error out"=w393:errorcluster)  [unwired: 9 in]
            n110 = Compound Arithmetic op=AND(w389, invert w387) -> (w388:bool)
            n111 = case shown="True" w388 {
              tunnel: w395 -> [w404 w413]
              tunnel: [w404 w412] -> w394
              tunnel: w392 -> [_ w409]
              tunnel: w393 -> [w402 w411]
              tunnel: [w401 w411] -> w397
              tunnel: [path "" w409] -> w384
              tunnel: [Picture_FGV_commands."No Action" ("Panel Picture Command") Picture_FGV_commands."Set Update Picture" ("Panel Picture Command")] -> w383
              tunnel: w386 -> [w399 w407]
              tunnel: [w399 w405] -> w385
              frame False {
                n112 = call <vilib>:"Clear Errors.vi"("error in (no error)"=w402) -> ("error out"=w401:errorcluster)  [unwired: 6 in]
              }
              frame True {
                n113 = Strip Path(path=w409) -> (name=w410:string)  [unwired: 1 out]
                n114 = Bundle By Name(cluster=w407, "IPF modified"=TRUE) -> (w405:T23)
                n115 = Bundle By Name(cluster=w413, "CAD Picture File"=w410) -> (w412:T19)
              }
            }
            n116 = call "Panel Picture FGV.vi"("Panel Picture Command"=w383, "Panel Picture path in"=w384) -> ()  [unwired: 12 in, 2 out]
          }
          event "Delete CAD Picture": Value Change {
            n117 = event-data() -> ()  [unwired: 1 in, 1 out]
            n118 = call "Panel Picture FGV.vi"("Panel Picture Command"=Picture_FGV_commands."Set Delete Picture", "Panel Picture path in"=path "") -> ()  [unwired: 12 in, 2 out]
            n119 = Bundle By Name(cluster=w420, "IPF modified"=TRUE) -> (w419:T23)
            n120 = Bundle By Name(cluster=w422, "CAD Picture File"="") -> (w421:T19)
          }
          event "butSave": Value Change {
            n121 = event-data() -> ()  [unwired: 1 in, 1 out]
            n122 = call "Save inspection prog  to IPF.vi"("Programming Data in"=w437, "Set Initial flag"=FALSE, "APG Config"=w427, "data in"=w436, "error in"=w438) -> ("Programming Data out"=w429:T23, "data out"=w435:T19, "error out"=w433:errorcluster)  [unwired: 8 in]
            n123 = call "Panel Picture FGV.vi"("Panel Picture Command"=Picture_FGV_commands."Get Picture action") -> ("Action"=w432:T34, "Panel Picture path out"=w431:path)  [unwired: 13 in]
            n124 = case shown="\"Delete Picture\"" w432 {
              tunnel: w433 -> [w444 w457 w460]
              tunnel: w431 -> [w441 _ _]
              tunnel: [w443 w448 w460] -> w430
              tunnel: w429 -> [w442 w452 _]
              tunnel: w427 -> [w440 w451 _]
              frame "Update Picture" {
                n125 = Build Array(file_types."CAD Picture" ("Descriptions")) -> (w445:T28[])
                n126 = call "Pack files.vi"("File type[]"=w445, "Programming Data In"=w442, "TCF/CAD Picture file"=w441, "APG Config"=w440, "error in (no error)"=w444) -> ("error out"=w443:errorcluster)  [unwired: 9 in, 1 out]
              }
              frame "Delete Picture" {
                n127 = Unbundle By Name(w451) -> ("IPF Folder"=w450:path)
                n128 = Unbundle By Name(w452) -> ("Programming Files.IPF temp folder"=w456:path)
                n129 = Strip Path(path=w456) -> (name=w455:string)  [unwired: 1 out]
                n130 = Build Path(base path=w450, name or relative path=w455) -> (appended path=w454:path)
                n131 = call-poly <userlib>:"Convert File Extension__ogtk.vi"("new ending (none)"="tar", "file name"=w454) -> ("new filename"=w447:path)  [unwired: 1 out]
                n132 = Build Array(file_types."CAD Picture" ("Descriptions")) -> (w458:T28[])
                n133 = call "Delete files.vi"("error in (no error)"=w457, "File type[]"=w458, "a3Di  tar file"=w447) -> ("error out"=w449:errorcluster)  [unwired: 7 in, 1 out]
                n134 = call "clean tar.vi"("tar file"=w447, "error in (no error)"=w449) -> ("error out"=w448:errorcluster)  [unwired: 12 in, 1 out]
              }
              frame "No Action" {
              }
            }
          }
          event Timeout {
            n135 = event-data() -> ()  [unwired: 1 in, 3 out]
          }
          event "butReload": Value Change {
            n136 = event-data() -> ()  [unwired: 1 in, 1 out]
            n137 = Unbundle By Name(w488) -> ("Programming Files.IPF temp folder"=w469:path)
            n138 = Unbundle By Name(w468) -> ("IPF Folder"=w474:path)
            n139 = Strip Path(path=w469) -> (name=w473:string)  [unwired: 1 out]
            n140 = Build Path(base path=w474, name or relative path=w473) -> (appended path=w472:path)
            n141 = Build Array(file_types."Inspection Prog" ("IPF File")) -> (w484:T28[])
            n142 = call "Unpack files.vi"("IPF files[]"=w484, "APG Config"=w468, "IPF cmd"=IPF_cmd."Edit IPF", "Destination folder"=w469, "error in (no error)"=w483) -> ("error out"=w481:errorcluster)  [unwired: 10 in]
            n143 = call-poly <userlib>:"Convert File Extension__ogtk.vi"("new ending (none)"="tar", "file name"=w472) -> ("new filename"=w470:path)  [unwired: 1 out]
            n144 = call "Inspection Program Read.vi"("error in (no error)"=w481, "ISP folder"=w469) -> ("error out"=w480:errorcluster, "data out"=w476:T19)  [unwired: 8 in]
            n145 = call "Picture file exists in Tar.vi"("a3Di  tar file"=w470, "error in (no error)"=w480) -> ("CAD Picture"=w477:string, "error out"=w478:errorcluster)  [unwired: 11 in, 1 out]
            n146 = Bundle By Name(cluster=w476, "CAD Picture File"=w477) -> (w475:T19)
            n147 = disable-structure shown="Enabled" {
              disable-tunnel: w469 -> [w494 _]
              disable-tunnel: [w493 w495] -> w486
              disable-tunnel: w475 -> [_ w496]
              frame Disabled {
                n148 = Strip Path(path=w494) -> (name=w493:string)  [unwired: 1 out]
              }
              frame Enabled {
                n149 = Unbundle By Name(w496) -> ("Program Name"=w495:string)
              }
            }
            n150 = Format Into String(format string="Program Inspection file %s loaded", error in=w478, w486) -> (resulting string=w490:string, error out=w479:errorcluster)  [unwired: 1 in]
            n151 = One Button Dialog(message=w490) -> ()  [unwired: 1 in, 1 out]
            n152 = Bundle By Name(cluster=w488, "IPF modified"=FALSE ("IPF saved")) -> (w487:T23)
          }
          event Value Change {
            n153 = event-data() -> ()  [unwired: 1 in, 1 out]
            n154 = control-ref of="This VI"() -> (w507:refnum<vi>)
            n155 = control-ref of="Checking results"() -> (w506:refnum<vi>)
            n156 = call "Debug main.vi"("Programming Data"=w508, "APG Config"=w505, "Dongle Fitted event Refnum in"=w504, "Edit IPFVI"=w507, "Checking results"=w506, "error in"=w509) -> ("Dongle fitted"=w497:bool, "error out"=w500:errorcluster)  [unwired: 12 in]
            n157 = case shown="False" w497 {
              tunnel: w500 -> [w513 w515]
              tunnel: [w512 w515] -> w499
              tunnel: w498 -> [w511 _]
              frame False {
                n158 = control-ref of="This VI"() -> (w514:refnum<vi>)
                n159 = call "Close subVI Vi when mainVI is active.vi"("error in (no error)"=w513, "Sub Vi ref"=w514, "Parent VI ref"=w511) -> ("error out"=w512:errorcluster)  [unwired: 8 in]
              }
              frame True {
              }
            }
            n160 = Select(t=state."Wait for user input" ("state"), s=w497, f=state."exit" ("state")) -> (s? t:f=w501:T24)
          }
          event Value Change {
            n161 = event-data() -> ()  [unwired: 1 in, 6 out]
            n162 = call "Set Robot Scan Direction.vi"("Scan Direction"=enum32{"X", "Y", "X and Y"}."X" ("Robot Scan Direction"), "Scan Params"="Scan Params") -> ("Scan Params"=w522:T15[])  [unwired: 9 in]
            n163 = Bundle By Name(cluster=w527, "Scan Params[]"=w522) -> (w526:T19)
            n164 = Bundle By Name(cluster=w519, "IPF modified"=TRUE ("IPF saved")) -> (w518:T23)
          }
          event "Robot Scan Direction": Value Change {
            n165 = event-data() -> ()  [unwired: 1 in, 6 out]
            n166 = Unbundle By Name(w534) -> ("Scan Params[]"=w533:T15[])
            n167 = call "Get Robot Scan Direction.vi"("Scan Params[]"=w533) -> ("Scan Params"=w535:T15)  [unwired: 9 in, 1 out]
            n168 = call "Set Robot Scan Direction.vi"("Scan Direction"="Robot Scan Direction", "Scan Params"=w535) -> ("Scan Params"=w538:T15[])  [unwired: 9 in]
            n169 = Bundle By Name(cluster=w534, "Scan Params[]"=w538) -> (w537:T19)
            n170 = Bundle By Name(cluster=w531, "IPF modified"=TRUE ("IPF saved")) -> (w530:T23)
          }
          event Value Change {
            n171 = event-data() -> ()  [unwired: 1 in, 6 out]
            n172 = Unbundle By Name("Panel Parameters") -> ("Name"=w550:string, "Pos & Rot"=w549:T8)
            n173 = Bundle By Name(cluster=w552, "Panel Params.Name"=w550, "Panel Params.Pos & Rot"=w549) -> (w548:T19)
            n174 = Bundle By Name(cluster=w544, "IPF modified"=TRUE ("IPF saved")) -> (w543:T23)
          }
          event Value Change {
            w583 = FALSE ("insert")
            n175 = event-data() -> ("OldVal"=w576:T11, "NewVal"=w559:T11)  [unwired: 1 in]
            n176 = Not Equal?(x=w576, y=w559) -> (x != y?=w577:T35)
            n177 = for {
              tunnel: w577 -> [w609] mode=indexing
              tunnel: [w608] -> w578
              tunnel: [w610] -> w579
              tunnel: [w611] -> w573
              i -> [w611]
              stop <- w607 stop-if-true
              n178 = Unbundle By Name(w609) -> ("insert"=w608:bool, "delete"=w610:bool)
              n179 = Or(x=w608, y=w610) -> (x .or. y?=w607:bool)
            }
            n180 = Index Array(array=w559, index=w573) -> (element=w581:T31)
            n181 = Bundle By Name(cluster=w581, "insert"=w583, "delete"=w583) -> (w582:T31)
            n182 = Replace Array Subset(array=w559, new element=w582, index=w573) -> (w575:T11)
            n183 = Build Array(w578, w579) -> (w580:bool[])
            n184 = Boolean Array To Number(Boolean array=w580) -> (number=w574:u32)
            n185 = case shown="2" w574 {
              tunnel: w573 -> [_ w595 w596]
              tunnel: [w590 w594 w600] -> w567
              tunnel: w575 -> [w590 w593 w606]
              frame 0, Default {
                # "Do nothing"
              }
              frame 1 {
                # "Insert new  entry to PCB List"
                n186 = Index Array(array=w593, index=-1) -> (element=w591:T31)
                n187 = Insert Into Array(array=w593, index=w595, new element=w591) -> (w594:T11)
              }
              frame 2 {
                # "Delete entry from PCB List"
                n188 = Delete From Array(array=w606, index=w596) -> (array with subset deleted=w600:T11)  [unwired: 1 in, 1 out]
                n189 = property on="PCBs List" class="Arr"("Value"=w600) -> ("Index Values"=w599:u32[])  [unwired: 2 in, 2 out]
                n190 = Array Size(array=w600) -> (size(s)=w604:i32)
                n191 = To Unsigned Long Integer(number=w604) -> (unsigned 32bit integer=w602:u32)
                n192 = Index Array(array=w599) -> (element=w598:u32)  [unwired: 1 in]
                n193 = Less?(x=w598, y=w602) -> (x < y?=w603:bool)
                n194 = Decrement(x=w602) -> (x-1=w601:u32)
                n195 = Select(t=w598, s=w603, f=w601) -> (s? t:f=w605:u32)
                n196 = Build Array(w605) -> (w597:u32[])
                n197 = property on="PCBs List" class="Arr"("Index Values"=w597) -> ()  [unwired: 2 in, 2 out]
              }
            }
            n198 = Bundle By Name(cluster=w556, "IPF modified"=TRUE ("IPF saved")) -> (w555:T23)
            n199 = Empty Array?(array=w567) -> (empty?=w570:bool)
            n200 = Select(t=T27."Disabled and Grayed Out" ("Disabled"), s=w570, f=T27."Enabled" ("Disabled")) -> (s? t:f=w569:T27)
            n201 = Unbundle By Name(T20 {"Name"="", "Pos & Rot"={"X"=0.0, "Y"=0.0, "Z"=0.0, "rotation"=0.0}, "PCBs List"=[], "PCB BarCode Params"=[], "Scan Type"=FALSE} ("Panel Params")) -> ("PCBs List"=w563:cluster{"PCB Params":T12}[])
            n202 = property on="insert" class="Bool"("DisabledEnum"=w569) -> ()  [unwired: 2 in, 2 out]
            n203 = Index Array(array=w563) -> (element=w562:cluster{"PCB Params":T12})  [unwired: 1 in]
            n204 = for {
              tunnel: w567 -> [w589] mode=indexing
              tunnel: [w586] -> w566 mode=indexing
              tunnel: w562 -> [w585]
              tunnel: [w584] -> w560 mode=indexing
              n205 = Unbundle By Name(w589) -> ("PCB Params.Name"=w588:string, "PCB Params.Pos & Rot"=w587:T8, "Barcode\nReader"=w584:cluster{"ID":T13})
              n206 = Bundle By Name(cluster=w585, "PCB Params.Name"=w588, "PCB Params.Pos & Rot"=w587) -> (w586:cluster{"PCB Params":T12})
            }
            n207 = Bundle By Name(cluster=w561, "Panel Params.PCBs List"=w566, "Panel Params.PCB BarCode Params"=w560) -> (w565:T19)
          }
          event "Fiducial List": Value Change {
            w636 = FALSE ("insert")
            # "If array is empty prevent delete button being pressed"
            n208 = event-data() -> ("OldVal"=w631:T10, "NewVal"=w630:T10)  [unwired: 1 in]
            n209 = Not Equal?(x=w631, y=w630) -> (x != y?=w632:T36)
            n210 = for {
              tunnel: w632 -> [w658] mode=indexing
              tunnel: [w659] -> w633
              tunnel: [w660] -> w634
              tunnel: [w661] -> w629
              i -> [w661]
              stop <- w662 stop-if-true
              n211 = Unbundle By Name(w658) -> ("insert"=w659:bool, "delete"=w660:bool)
              n212 = Or(x=w659, y=w660) -> (x .or. y?=w662:bool)
            }
            n213 = Index Array(array=w630, index=w629) -> (element=w637:T32)
            n214 = Bundle By Name(cluster=w637, "insert"=w636, "delete"=w636) -> (w635:T32)
            n215 = Build Array(w633, w634) -> (w638:bool[])
            n216 = Replace Array Subset(array=w630, new element=w635, index=w629) -> (w627:T10)
            n217 = Boolean Array To Number(Boolean array=w638) -> (number=w628:u32)
            n218 = Bundle By Name(cluster=w616, "IPF modified"=TRUE ("IPF saved")) -> (w615:T23)
            n219 = case shown="2" w628 {
              tunnel: w629 -> [_ w646 w657]
              tunnel: [w641 w645 w649] -> w621
              tunnel: w627 -> [w641 w644 w656]
              frame 0, Default {
                # "Do nothing"
              }
              frame 1 {
                # "Insert new entry to Fiducial List"
                n220 = Index Array "get default element"(array=w644, index=-1) -> (element=w642:T32)
                n221 = Insert Into Array(array=w644, index=w646, new element=w642) -> (w645:T10)
              }
              frame 2 {
                # "Delete entry from fiducial List"
                n222 = Delete From Array(array=w656, index=w657) -> (array with subset deleted=w649:T10)  [unwired: 1 in, 1 out]
                n223 = Array Size(array=w649) -> (size(s)=w655:i32)
                n224 = property on="Fiducial List" class="Arr"("Value"=w649) -> ("Index Values"=w648:u32[])  [unwired: 2 in, 2 out]
                n225 = To Unsigned Long Integer(number=w655) -> (unsigned 32bit integer=w654:u32)
                n226 = Index Array(array=w648) -> (element=w647:u32)  [unwired: 1 in]
                n227 = Less?(x=w647, y=w654) -> (x < y?=w653:bool)
                n228 = Decrement(x=w654) -> (x-1=w652:u32)
                n229 = Select(t=w647, s=w653, f=w652) -> (s? t:f=w651:u32)
                n230 = Build Array(w651) -> (w650:u32[])
                n231 = property on="Fiducial List" class="Arr"("Index Values"=w650) -> ()  [unwired: 2 in, 2 out]
              }
            }
            n232 = for {
              tunnel: w621 -> [w640] mode=indexing
              tunnel: [w639] -> w620 mode=indexing
              n233 = Unbundle By Name(w640) -> ("Fiducial"=w639:T33)
            }
            n234 = Empty Array?(array=w621) -> (empty?=w624:bool)
            n235 = Select(t=T27."Disabled and Grayed Out" ("Disabled"), s=w624, f=T27."Enabled" ("Disabled")) -> (s? t:f=w613:T27)
            n236 = Bundle By Name(cluster=w622, "Inspection Data.Fiducial List"=w620) -> (w623:T19)
            n237 = property on="delete" class="Bool"("DisabledEnum"=w613) -> ()  [unwired: 2 in, 2 out]
          }
          event Value Change {
            n238 = event-data() -> ()  [unwired: 1 in, 6 out]
            n239 = Bundle By Name(cluster=w666, "IPF modified"=TRUE ("IPF saved")) -> (w665:T23)
            n240 = Bundle By Name(cluster=w672, "Description"="Description") -> (w670:T19)
          }
          event "Start Conversion ODB++": Value Change {
            n241 = event-data() -> ()  [unwired: 1 in, 1 out]
            n242 = control-ref of="Debug Results Button"() -> (w681:refnum<vi>)
            n243 = control-ref of="insert"() -> (w680:refnum<vi>)
            n244 = control-ref of="Update TCF button"() -> (w679:refnum<vi>)
            n245 = control-ref of="delete"() -> (w678:refnum<vi>)
            n246 = control-ref of="Test Coverage Button"() -> (w677:refnum<vi>)
            n247 = control-ref of="Generate Library button"() -> (w673:refnum<vi>)
            n248 = control-ref of="Scan Params"() -> (w674:refnum<vi>)
            n249 = control-ref of="PCBs List"() -> (w676:refnum<vi>)
            n250 = control-ref of="Fiducial List"() -> (w675:refnum<vi>)
            n251 = Bundle By Name(cluster=T30 {"Debug Results Button"=refnum, "insert"=refnum, "Update TCF button"=refnum, "delete"=refnum, "Test Coverage Button"=refnum, "PCBs List"=refnum, "Fiducial List"=refnum, "Scan Params"=refnum, "Generate Library Button"=refnum} ("FP ctrl references"), "Debug Results Button"=w681, "insert"=w680, "Update TCF button"=w679, "delete"=w678, "Test Coverage Button"=w677, "PCBs List"=w676, "Fiducial List"=w675, "Scan Params"=w674, "Generate Library Button"=w673) -> (w682:T30)
            n252 = call "import ODB.vi"("Dongle Fitted event Refnum in"=w691, "Programming Data"=w694, "APG Config"=w697, "Data"=w693, "error in"=w698, "Edit VI"=w695, "FP ctrl references"=w682) -> ("Programming Data out"=w696:T23, "Data out"=w699:T19, "Dongle fitted"=w684:bool, "APG Config"=w692:T6, "error out"=w687:errorcluster)  [unwired: 8 in]
            n253 = case shown="True" w684 {
              tunnel: w687 -> [w702 w704]
              tunnel: [w701 w704] -> w686
              tunnel: w685 -> [w700 _]
              frame False {
                n254 = control-ref of="This VI"() -> (w703:refnum<vi>)
                n255 = call "Close subVI Vi when mainVI is active.vi"("error in (no error)"=w702, "Sub Vi ref"=w703, "Parent VI ref"=w700) -> ("error out"=w701:errorcluster)  [unwired: 8 in]
              }
              frame True {
              }
            }
            n256 = Select(t=state."Wait for user input" ("state"), s=w684, f=state."exit" ("state")) -> (s? t:f=w688:T24)
          }
          event Value Change {
            n257 = event-data() -> ()  [unwired: 1 in, 1 out]
            n258 = call-poly <vilib>:"Set Cursor.vi"("error in (no error)"=w717, "icon"=u16 2) -> ("error out"=w716:errorcluster)  [unwired: 8 in, 1 out]
            n259 = call "Generate Library from TCF.vi"("APG Config"=w707, "Inspection Data"=w718, "error in"=w716) -> ("APG Config"=w706:T6, "Library successfully generated"=w708:bool, "Library Generation cancelled"=w709:bool, "error out"=w714:errorcluster)  [unwired: 9 in]
            n260 = case shown="True" w709 {
              tunnel: [w722 "Library Generation cancelled" ("message")] -> w710
              tunnel: w708 -> [w721 _]
              frame False {
                n261 = case shown="False" w721 {
                  tunnel: ["Failed to generate Library from TCF\nCheck Library file and  folder settings" ("message") "Library successfully created from TCF" ("message")] -> w722
                  frame False {
                  }
                  frame True {
                  }
                }
              }
              frame True {
              }
            }
            n262 = call-poly <vilib>:"Set Cursor.vi"("error in (no error)"=w714, "icon"=u16 0) -> ("error out"=w712:errorcluster)  [unwired: 8 in, 1 out]
            n263 = flat-sequence {
              tunnel: w712 -> [w727]
              tunnel: [w727] -> w711
              tunnel: w710 -> [w726]
              frame #0 {
                n264 = One Button Dialog(message=w726) -> ()  [unwired: 1 in, 1 out]
              }
            }
          }
          event Value Change {
            n265 = event-data() -> ()  [unwired: 1 in, 1 out]
            n266 = call "Four Button Dialog.vi"("Left Button Text"="Device Library", "Message"="TCF Update Method", "Centre Left Button Text"="Manual Update", "Centre Right Button Text"="BOM List/TCF PartNo", "Right Button Text"="Cancel") -> ("Which Button?"=w734:T37)  [unwired: 9 in, 1 out]
            n267 = case shown="\"Centre Right\"" w734 {
              tunnel: w728 -> [w760 w778 w785 w789]
              tunnel: w744 -> [w759 w776 w784 w788]
              tunnel: [w750 w776 w784 w788] -> w746
              tunnel: w745 -> [w758 w775 w779 w787]
              tunnel: [w756 w777 w780 w789] -> w739
              tunnel: [w751 w775 w779 w787] -> w747
              tunnel: w743 -> [w752 w774 w782 _]
              tunnel: [w749 w773 w783 TRUE ("Dongle fitted")] -> w736
              tunnel: w735 -> [_ _ w781 _]
              frame "Left" {
                n268 = call "TCF Update.vi"("Programming Data In"=w759, "ODB import"=FALSE, "Dongle Fitted event Refnum in"=w752, "APG Config"=w758, "error in (no error)"=w760) -> ("Programming Data Out"=w753:T23, "Dongle fitted"=w749:bool, "APG Config"=w755:T6, "error out"=w754:errorcluster)  [unwired: 6 in, 1 out]
                n269 = case shown="True" w749 {
                  tunnel: [w763 w769] -> w756
                  tunnel: w755 -> [w761 w765]
                  tunnel: w754 -> [w763 w768]
                  tunnel: w753 -> [w762 w764]
                  tunnel: [w761 w765] -> w751
                  tunnel: [w762 w764] -> w750
                  frame False {
                  }
                  frame True {
                    n270 = call "Get TCF from temp folder.vi"("error in (no error)"=w768, "Programming Data"=w764) -> ("error out"=w767:errorcluster, "TCF file"=w766:path)  [unwired: 8 in]
                    n271 = Build Array(file_types."TCF" ("Descriptions")) -> (w772:T28[])
                    n272 = call "Pack files.vi"("File type[]"=w772, "TCF in scan tar"=FALSE, "Programming Data In"=w764, "TCF/CAD Picture file"=w766, "APG Config"=w765, "error in (no error)"=w767) -> ("error out"=w769:errorcluster)  [unwired: 8 in, 1 out]
                  }
                }
              }
              frame "Centre Left" {
                n273 = call "TCF Manual Update.vi"("Programming Data In"=w776, "Dongle Fitted event Refnum in"=w774, "APG Config"=w775, "error in (no error)"=w778) -> ("Dongle fitted"=w773:bool, "error out"=w777:errorcluster)  [unwired: 10 in]
              }
              frame "Centre Right" {
                n274 = call "Update TCF with BOM.vi"("Programming Data In"=w784, "VI ref in"=w781, "Dongle Fitted event Refnum in"=w782, "APG Config"=w779, "error in (no error)"=w785) -> ("Dongle fitted"=w783:bool, "error out"=w780:errorcluster)  [unwired: 9 in]
              }
              frame "Right", "Panel Close" {
              }
            }
            n275 = case shown="False" w736 {
              tunnel: w739 -> [w792 w794]
              tunnel: [w791 w794] -> w738
              tunnel: w737 -> [w790 _]
              frame False {
                n276 = control-ref of="This VI"() -> (w793:refnum<vi>)
                n277 = call "Close subVI Vi when mainVI is active.vi"("error in (no error)"=w792, "Sub Vi ref"=w793, "Parent VI ref"=w790) -> ("error out"=w791:errorcluster)  [unwired: 8 in]
              }
              frame True {
              }
            }
            n278 = Select(t=state."Wait for user input" ("state"), s=w736, f=state."exit" ("state")) -> (s? t:f=w740:T24)
          }
          event Value Change {
            n279 = event-data() -> ()  [unwired: 1 in, 1 out]
            n280 = call "Display PCB coverage.vi"("Inspection Data"=w803, "Dongle Fitted event Refnum in"=w802, "error in (no error)"=w804) -> ("Dongle fitted"=w795:bool, "error out"=w798:errorcluster)  [unwired: 11 in]
            n281 = case shown="False" w795 {
              tunnel: w798 -> [w809 w811]
              tunnel: [w808 w811] -> w796
              tunnel: w797 -> [w807 _]
              frame False {
                n282 = control-ref of="This VI"() -> (w810:refnum<vi>)
                n283 = call "Close subVI Vi when mainVI is active.vi"("error in (no error)"=w809, "Sub Vi ref"=w810, "Parent VI ref"=w807) -> ("error out"=w808:errorcluster)  [unwired: 8 in]
              }
              frame True {
              }
            }
            n284 = Select(t=state."Wait for user input" ("state"), s=w795, f=state."exit" ("state")) -> (s? t:f=w799:T24)
          }
          event "Initial Scan Button": Value Change {
            n285 = event-data() -> ()  [unwired: 1 in, 1 out]
            n286 = Unbundle By Name(w818) -> ("Scan Params[]"=w815:T15[])
            n287 = for {
              tunnel: w815 -> [w826] mode=indexing
              tunnel: "Initial Scan Button" -> [w825]
              tunnel: [w824] -> w813 mode=indexing
              n288 = Bundle By Name(cluster=w826, "Initial scan"=w825) -> (w824:T15)
            }
            n289 = Bundle By Name(cluster=w818, "Scan Params[]"=w813) -> (w817:T19)
            n290 = Bundle By Name(cluster=w820, "IPF modified"=TRUE ("IPF saved")) -> (w821:T23)
          }
          event "Product Code": Value Change {
            n291 = event-data() -> ()  [unwired: 1 in, 1 out]
            n292 = Search and Replace String(input string="Product Code", search string="\n", replace string="") -> (result string=w828:string)  [unwired: 5 in, 3 out]
            n293 = Bundle By Name(cluster=w840, "IPF modified"=TRUE ("IPF saved")) -> (w839:T23)
            n294 = Bundle By Name(cluster=w837, "Product Code"=w828) -> (w836:T19)
            n295 = property on="Product Code" class="Str"(error in=w830, "Value"=w828, "Key Focus"=TRUE) -> (error out=w829:errorcluster)  [unwired: 1 in, 1 out]
          }
          event "Side ID": Value Change {
            n296 = event-data() -> ()  [unwired: 1 in, 1 out]
            n297 = Bundle By Name(cluster=w844, "Side ID"="Side ID") -> (w843:T19)
            n298 = Bundle By Name(cluster=w848, "IPF modified"=TRUE ("IPF saved")) -> (w847:T23)
          }
        }
      }
      frame "exit" {
        # "Exit application"
      }
    }
    n299 = Unbundle By Name(w38) -> ("Side ID"=w24:string, "Product Code"=w25:string, "CAD Picture File"=→"Panel Picture File":string, "Program Name"=→"Program Name":string, "Scan Params[]"=w43:T15[], "Description"=w53:string, "Control File Relative Path"=w35:path, "PCB Outline File"=w33:path, "Inspection Data"=w52:T22, "Panel Params"=w51:T20)
    n300 = Unbundle By Name(w59) -> ("status"=w58:bool)
    n301 = control-ref of="delete"() -> (w29:refnum<vi>)
    n302 = control-ref of="insert"() -> (w48:refnum<vi>)
    n303 = Unbundle By Name(w38) -> ("Program Name"=w28:string)
    n304 = Or(x=w58, y=w57) -> (x .or. y?=w60:bool)
    n305 = call "Get Robot Scan Direction.vi"("Scan Params[]"=w43) -> ("Scan Direction"=w42:enum32{"X", "Y", "X and Y"}, "Scan Params"=w26:T15)  [unwired: 9 in]
    n306 = call "PCB list format to GUI.vi"("delete ref"=w48, "File Panal Params"=w51) -> ("GUI Panel & PCB Params"=w50:T38)  [unwired: 13 in]
    n307 = call "inspection data format to GUI.vi"("delete"=w29, "Inspection Data"=w52) -> ("Fiducial List"=w47:T39)  [unwired: 13 in]
    n308 = Strip Path(path=w33) -> (name=→"PCB Outline File":string)  [unwired: 1 out]
    n309 = Strip Path(path=w35) -> (name=→"Control File":string)  [unwired: 1 out]
    n310 = local write "Description"(w53) -> ()
    n311 = Unbundle By Name(w50) -> ("Panel Params"=w49:T14, "PCBs List"=w46:T11)
    n312 = local write "Robot Scan Direction"(w42) -> ()
    n313 = local write "Side ID"(w24) -> ()
    n314 = local write "Product Code"(w25) -> ()
    n315 = local write "Scan Params"(w26) -> ()
    n316 = Unbundle By Name(w26) -> ("Initial scan"=w27:bool)
    n317 = local write "Fiducial List"(w47) -> ()
    n318 = local write "Initial Scan Button"(w27) -> ()
    n319 = local write "Panel Parameters"(w49) -> ()
    n320 = local write "PCBs List"(w46) -> ()
  }
  "error out" <- w17
  "Program Name" <- w11
  "Dongle fitted" <- w1
